vi "TLB Native Dynamic Events ver 0.13e.vi"() -> ()   [LabVIEW 2018]
uses:
  Labview Training Phase 2/Enum Controls/States for Action Engine.ctl
  TLB Type Definitions/State Type Definitions, for 0.26g versions and later 2.ctl
  TLB Type Definitions/Intruction Type Definitions.ctl
  TLB Type Definitions/Encoder cluster.ctl
  TLB Type Definitions/PING CLUSTER.ctl
  <vilib>/Studica/Studica Toolkit/NavX/NavX.lvlib
  <vilib>/Studica/Studica Toolkit/Background/DIO Channel.ctl
  Underlying VI's/NavX VI/navX type def.ctl
  <vilib>/myRIO/Instrument Drivers/Utilities/Utilities.lvlib
  <vilib>/Studica/Studica Toolkit/Background/I2C Channel.ctl
  TLB Type Definitions/Vision cluster.ctl
  <vilib>/NI_Real-Time Target Support.lvlib
  TLB Type Definitions/Stepper cluster.ctl
  Experimental VI's/Archived VI's/MOTOR CONTROL NO PID Type Def.ctl
  Underlying VI's/I2C Master VI/I2C MASTER Type Def.ctl
  Underlying VI's/I2C Master VI/I2C_MASTER_WRITE_NEW Type Def.ctl
  Underlying VI's/Webcam FGV Low level ver/State control.ctl
  <vilib>/userdefined/High Color/IMAQdx.ctl
  Underlying VI's/I2C Master VI/Arduino_Interfacing.ctl
  TLB Type Definitions/Yaw Cluster.ctl
  Experimental VI's/Archived VI's/MOTOR CONTROL NO PID AE DATA ENTRY MODE Type def.ctl
  Experimental VI's/Archived VI's/MOTOR CONTROL NO PID AE DIRECTIONS type def.ctl
  Underlying VI's/Elasped Timer/Control.ctl
  TLB Type Definitions/Time cluster.ctl
  <vilib>/Utility/RT CPU Load.ctl
panel:
  out "Time up flag":bool
  out "Recognized object + Time up?":bool
  out "Speed & distance":T1
  out "Task selection":u8
  out "Object Center Coordinates":cluster{"x":sgl, "y":sgl}
  out "Object detection cluster":T2
  in  "Object recognition mode":enum16{"Ball", "Soap", "Gel", "Pipe", "None"}(ring)
  out "NavX Readings":T3
  out "Arduino Data":T4
  out "CPU loads":T5[](array[typedef]) {"ISR (%)" format="%#.2f"; "Idle (%)" format="%#.2f"; "Background (%)" format="%#.2f"; "Normal (%)" format="%#.2f"; "Above Normal (%)" format="%#.2f"; "High (%)" format="%#.2g"; "Timed Structures (%)" format="%#.2g"; "Time Critical (%)" format="%#.2g"; "Total (%)" format="%#.2g"}
  in  "Red LED":bool
  out "Detect?":bool
  out "TASK ENABLE":bool
  out "Rising Edge":bool
  in  "Green LED":bool
  out "Object detected?":bool
  out "I2C Error":errorcluster
  out "State Logic":T6=enum."Startup"
  out "elements":T7[](array[typedef])
  in  "STOP TASK":bool
  in  "OK Button":bool
  in  "STOP":bool
  out "error out":errorcluster
  out "Action Queue Items":i32
  out "State Logic Queue Items":i32
  out "Action Queues items":string[](array[string])=["Hardware reset", "Software reset", ""]
  out "Action State":string
  # "TLB FRAMEWORK STATUS"
  # "System Health Status Update"
  # "Test Programme written by Calvin Loke    Dated: 28 Aug 2019\nTest Programme revised by Dr Alex See   Dated 30 Aug 2019\n\nProgramme version:   TLB Native Dynamic Events ver 0.04b.vi"
  # "VISION"
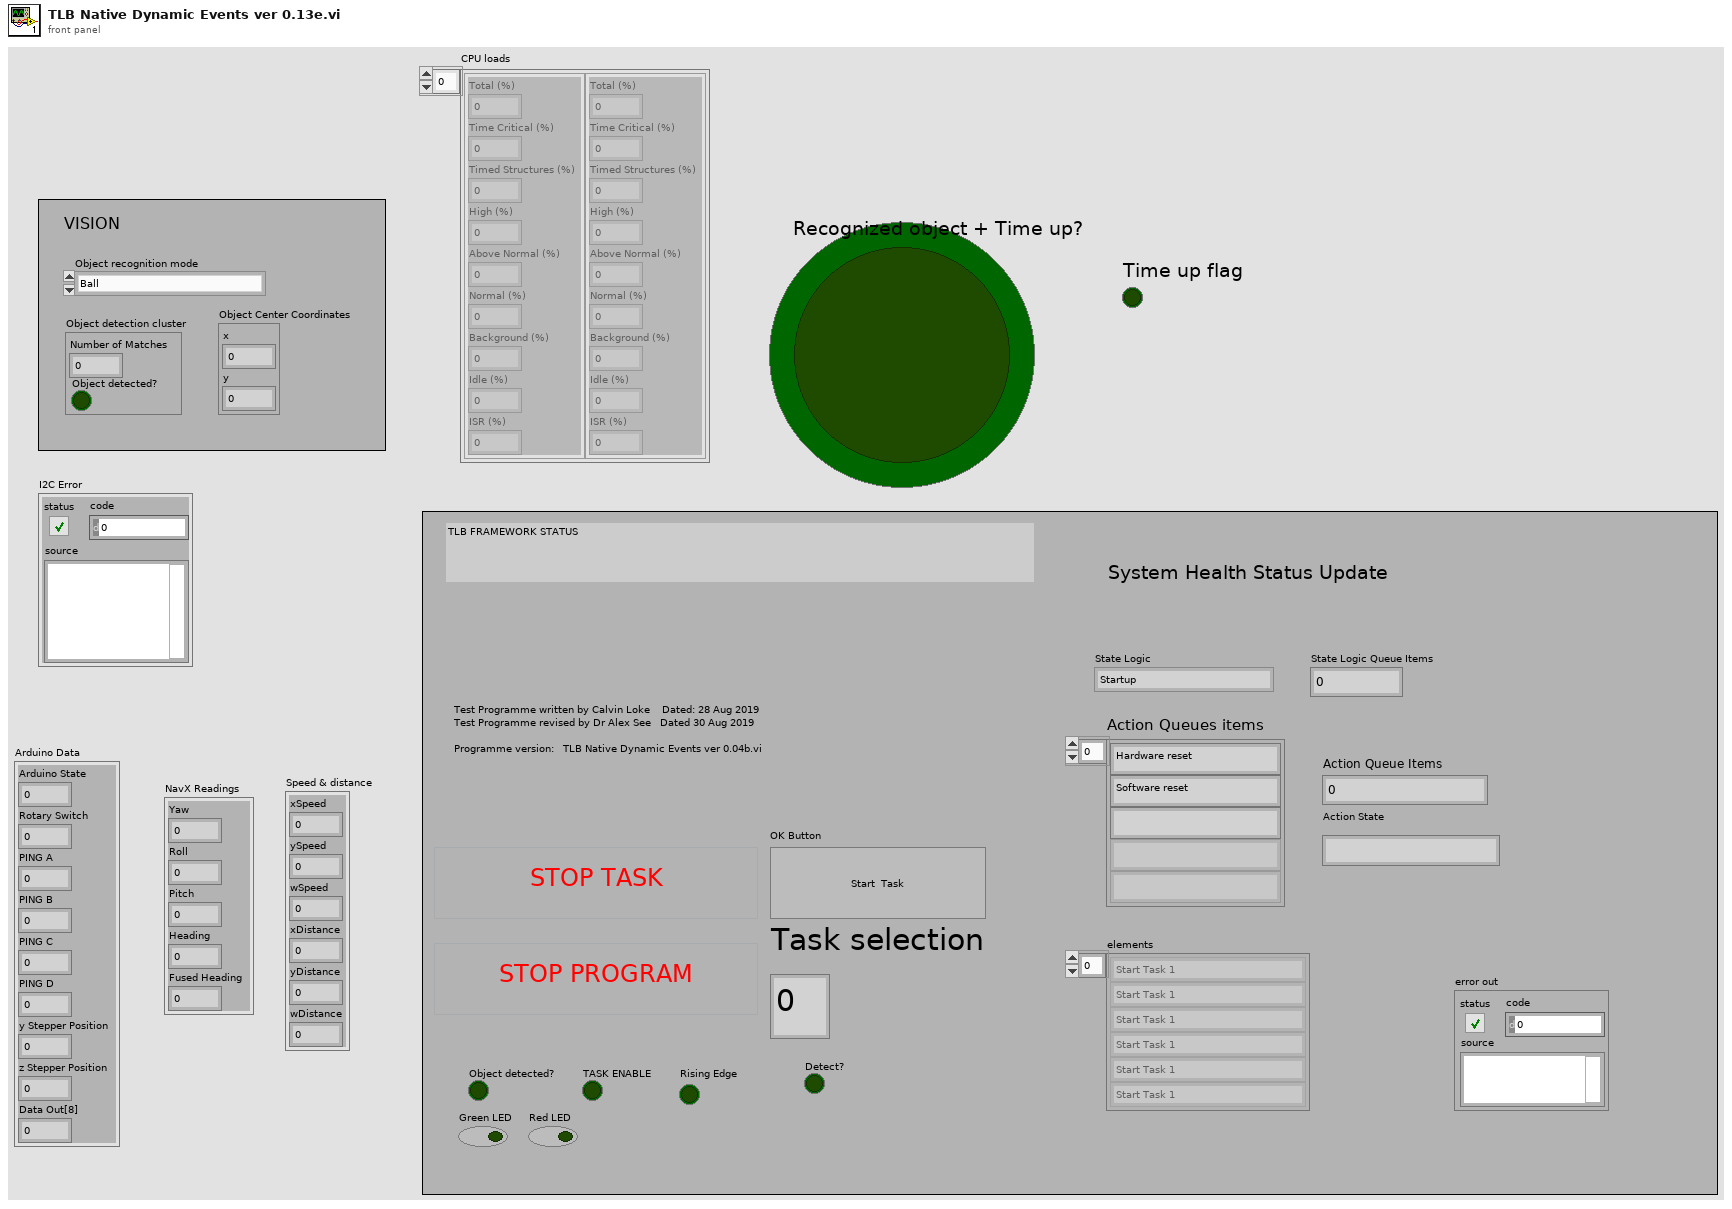
[diagram p1: front panel]
types:
  T1 = cluster{"xSpeed":dbl, "ySpeed":dbl, "wSpeed":dbl, "xDistance":dbl, "yDistance":dbl, "wDistance":dbl}
  T2 = cluster{"Number of Matches":i32, "Object detected?":bool}
  T3 = cluster{"Yaw":dbl, "Roll":dbl, "Pitch":dbl, "Heading":dbl, "Fused Heading":dbl}
  T4 = cluster{"Arduino State":u8, "Rotary Switch":u8, "PING A":u8, "PING B":u8, "PING C":u8, "PING D":u8, "y Stepper Position":u8, "z Stepper Position":u8, "Data Out[8]":u8}
  T5 = typedef "NI_Real-Time Target Support.lvlib/RT CPU Load.ctl" = cluster{"Total (%)":dbl, "Time Critical (%)":dbl, "Timed Structures (%)":dbl, "High (%)":dbl, "Above Normal (%)":dbl, "Normal (%)":dbl, "Background (%)":dbl, "Idle (%)":dbl, "ISR (%)":dbl}
  T6 = typedef "State Type Definitions, for 0.26g versions and later 2.ctl" = enum16{"None", "Startup", "Move to Angle", "True Stop", "Idle", "Shutdown", "Task 1A", "Task 1B", "Task 2:Raise Arm", "Task 2:Sensor Mode", "Task 2:Reverse Mode", "Task 3", "Task 4_A", "Task 4_B", "Task 4_C", "Task 4_D", "Task 5A", "Task 5B", "Task 5C", "Task 5D", "Task 5E: POSITION ARM", "Task 5F: ARM GRAB HEIGHT", "Task 5G: CLOSE CLAW", "Task 5H: RAISE ARM", "Task 6_A", "Task 6_B", "Task 7", "Task 8A: RAISE ARM", "Task 8B: MOVE TO BOX", "Task 8C: CAM BURST", "Task 8D: PROCESS IMAGE", "Task 8E: ROBOT ADJUST", "Task 8F: CAM BURST 2", "Task 8G: PROCESS IMAGE 2", "Task 8H: ARM ADJUST", "Task 8I: ARM GRAB HEIGHT", "Task 8J: CLOSE CLAW", "Task 8K: RAISE MY SWORD", "Task 9A: Raise Arm", "Task 9B: Rotate to Angle", "Task 9C: Detect Box", "Task 9D: MOVE FORWARD", "Task 9E: MOVE LEFT", "Task 9F: SCAN BOX", "Task 9G: MOVE RIGHT", "Task 9H: SCAN BOX 2", "Task 9I: ROTATE 90 CW", "Task 9J: FORWARD", "Task 9K: MOVE RIGHT", "Task 9L: SCAN BOX 3", "Task 9M: MOVE RIGHT", "Task 9N: SCAN BOX 4", "PENIS", "PENIS 2", "PENIS 3", "Task 9R: PROCESS COLOUR", "Task A1: Task 9 Open cam", "Task A2: Task 9 Move Arm", "Task A3: Task 9 Set Timer", "Task A4: Tasl 9 Capture images", "Task A5: Task 9 Close camera", "Task A6: Process Colour", "Task A7: Dispose Camera Buffer"}
  T7 = typedef "Intruction Type Definitions.ctl" = enum16{"None", "Start Task 1", "Start Task 2", "Start Task 3", "Start Task 4", "Start Task 5", "Start Task 6", "Start Task 7", "Start Task 8 - BALL", "Start Task 8 - Gel", "Start Task 8 - Pipe", "Start Task 8 - Soap", "Start Task 9", "Start Task A", "Start Task B", "Exit"}
  T8 = typedef "Time cluster.ctl" = cluster{"Time up flag":bool, "SET TIME TO CHECK":dbl}
  T9 = typedef "Yaw Cluster.ctl" = cluster{"Yaw":dbl, "Compass":dbl}
  T10 = typedef "Stepper cluster.ctl" = cluster{"y Stepper Position":u8, "z Stepper Position":u8}
  T11 = typedef "DIO Channel.ctl" = enum16{"Not Connected", "A/DIO1", "A/DIO2", "A/DIO3", "A/DIO4", "A/DIO5", "A/DIO6", "A/DIO7", "A/DIO13", "B/DIO1", "B/DIO2", "B/DIO3", "B/DIO4", "B/DIO5", "B/DIO6", "B/DIO7", "B/DIO13", "C/DIO0", "C/DIO1", "C/DIO2", "C/DIO3", "C/DIO4", "C/DIO5", "C/DIO6", "C/DIO7"}
  T12 = typedef "Vision cluster.ctl" = cluster{"Recognized Object":bool, "Object X coordinate":dbl, "Object Y coordinate":dbl}
  T13 = typedef "PING CLUSTER.ctl" = cluster{"PING_A":u8, "PING_B":u8, "PING_C":u8, "PING_D":u8}
  T14 = typedef "Encoder cluster.ctl" = cluster{"xDistance":dbl, "yDistance":dbl, "wDistance":dbl}
  T15 = cluster{"DIO Channel":T11, "FPGA VI Reference Out":refnum<k20>}
  T16 = typedef "MOTOR CONTROL NO PID AE DATA ENTRY MODE Type def.ctl" = enum16{"Initialize", "Reset Encoders", "Write to motors", "Read from Encoders"}
  T17 = typedef "navX type def.ctl" = enum16{"Get i2C reference", "Read Values", "Zero Yaw"}
  T18 = typedef "Arduino_Interfacing.ctl" = enum16{"Initialize", "Write to Arduino", "Read From Arduino"}
  T19 = typedef "I2C Channel.ctl" = enum16{"Not Connected", "A", "B"}
  T20 = typedef "States for Action Engine.ctl" = enum16{"Initialize", "Write", "Read"}
  T21 = cluster{"I2C Ref Out":cluster{"I2C Channel":T19, "FPGA VI Reference Out":refnum<k20>}, "Connected":bool, "Slave Address (7-bit)":u8, "Registry":u8[]}
  T22 = typedef "IMAQ Image.ctl" = refnum<image>
  T23 = typedef "State Type Definitions.ctl" = enum16{"None", "Startup", "Move to Angle", "True Stop", "Idle", "Shutdown", "Task 1", "Task 2:Raise Arm", "Task 2:Sensor Mode", "Task 2:Reverse Mode", "Task 3", "Task 4_A", "Task 4_B", "Task 4_C", "Task 4_D", "Task 5A: ARM CAM HEIGHT", "Task 5B: MOVE TO BOX", "Task 5C: CAM BURST", "Task 5D: PROCESS IMAGE", "Task 5E: POSITION ARM", "Task 5F: ARM GRAB HEIGHT", "Task 5G: CLOSE CLAW", "Task 5H: RAISE ARM", "Task 6_A", "Task 6_B", "Task 7", "Task 8A: RAISE ARM", "Task 8B: MOVE TO BOX", "Task 8C: CAM BURST", "Task 8D: PROCESS IMAGE", "Task 8E: ROBOT ADJUST", "Task 8F: CAM BURST 2", "Task 8G: PROCESS IMAGE 2", "Task 8H: ARM ADJUST", "Task 8I: ARM GRAB HEIGHT", "Task 8J: CLOSE CLAW", "Task 8K: RAISE MY SWORD", "Task 9A: Raise Arm", "Task 9B: Rotate to Angle", "Task 9C: Detect Box", "Task 9D: MOVE FORWARD", "Task 9E: MOVE LEFT", "Task 9F: SCAN IMAGE", "Task 9G: PROCESS COLOUR", "Task 9H: MOVE RIGHT", "Task 9I: SCAN IMAGE", "Task 9J: PROCESS COLOUR", "Task 9K: ROTATE 90 CW", "Task 9L: MOVE FORWARD", "Task 9M: MOVE RIGHT", "Task 9N: SCAN IMAGE", "Task 9O: PROCESS COLOUR", "Task 9P: MOVE RIGHT", "Task 9Q: SCAN IMAGE", "Task 9R: PROCESS COLOUR"}
  T24 = typedef "State Type Definitions.ctl" = enum16{"None", "Startup", "Move to Angle", "True Stop", "Idle", "Shutdown", "Task 1", "Task 2", "Task 3", "Task 4_A", "Task 4_B", "Task 4_C", "Task 5_A", "Task 5 _B", "Task 5_C", "Task 6_A", "Task 6_B", "Task 7", "Task 8", "Task 9", "Task A", "Task B"}
  T25 = typedef "MOTOR CONTROL NO PID AE DIRECTIONS type def.ctl" = enum16{"y-axis movement", "x-axis movement", "Rotate", "Stop"}
  T26 = typedef "Control.ctl" = enum16{"Start", "Pause", "Initialize"}
  T27 = typedef "I2C_MASTER_WRITE_NEW Type Def.ctl" = enum16{"Ultrasonic sensors", "Stepper origin", "zStepper 13.3k", "zStepper 13k", "zStepper 12k", "zStepper 11k", "zStepper 10k", "zStepper 9k", "zStepper 8k", "zStepper 7k", "zStepper 6k", "zStepper 5k", "zStepper 4k", "zStepper 3k", "zStepper 2k", "zStepper 1k", "zStepper 900", "zStepper 800", "zStepper 700", "zStepper 600", "zStepper 500", "zStepper 400", "zStepper 300", "zStepper 200", "zStepper 100", "zStepper 0", "yStepper control", "Open Claw", "Close Claw", "Soft Reset"}
  T28 = typedef "State control.ctl" = enum16{"Initialise", "Start camera", "Continuous Acquisition ", "Stop camera", "Dispose all"}
  T29 = typedef "IMAQdx.ctl" = refnum<k21>
  T30 = typedef "MOTOR CONTROL NO PID Type Def.ctl" = enum16{"Init", "Front Back", "Left Right", "Rotate", "Stop", "Latch"}
  T31 = typedef "I2C MASTER Type Def.ctl" = enum16{"Last State", "Mode 0", "Mode 1", "Mode 2", "Mode 3", "Mode 4", "Mode 5", "Mode 6", "Mode 7", "Mode 8", "Mode 9", "Mode 10"}
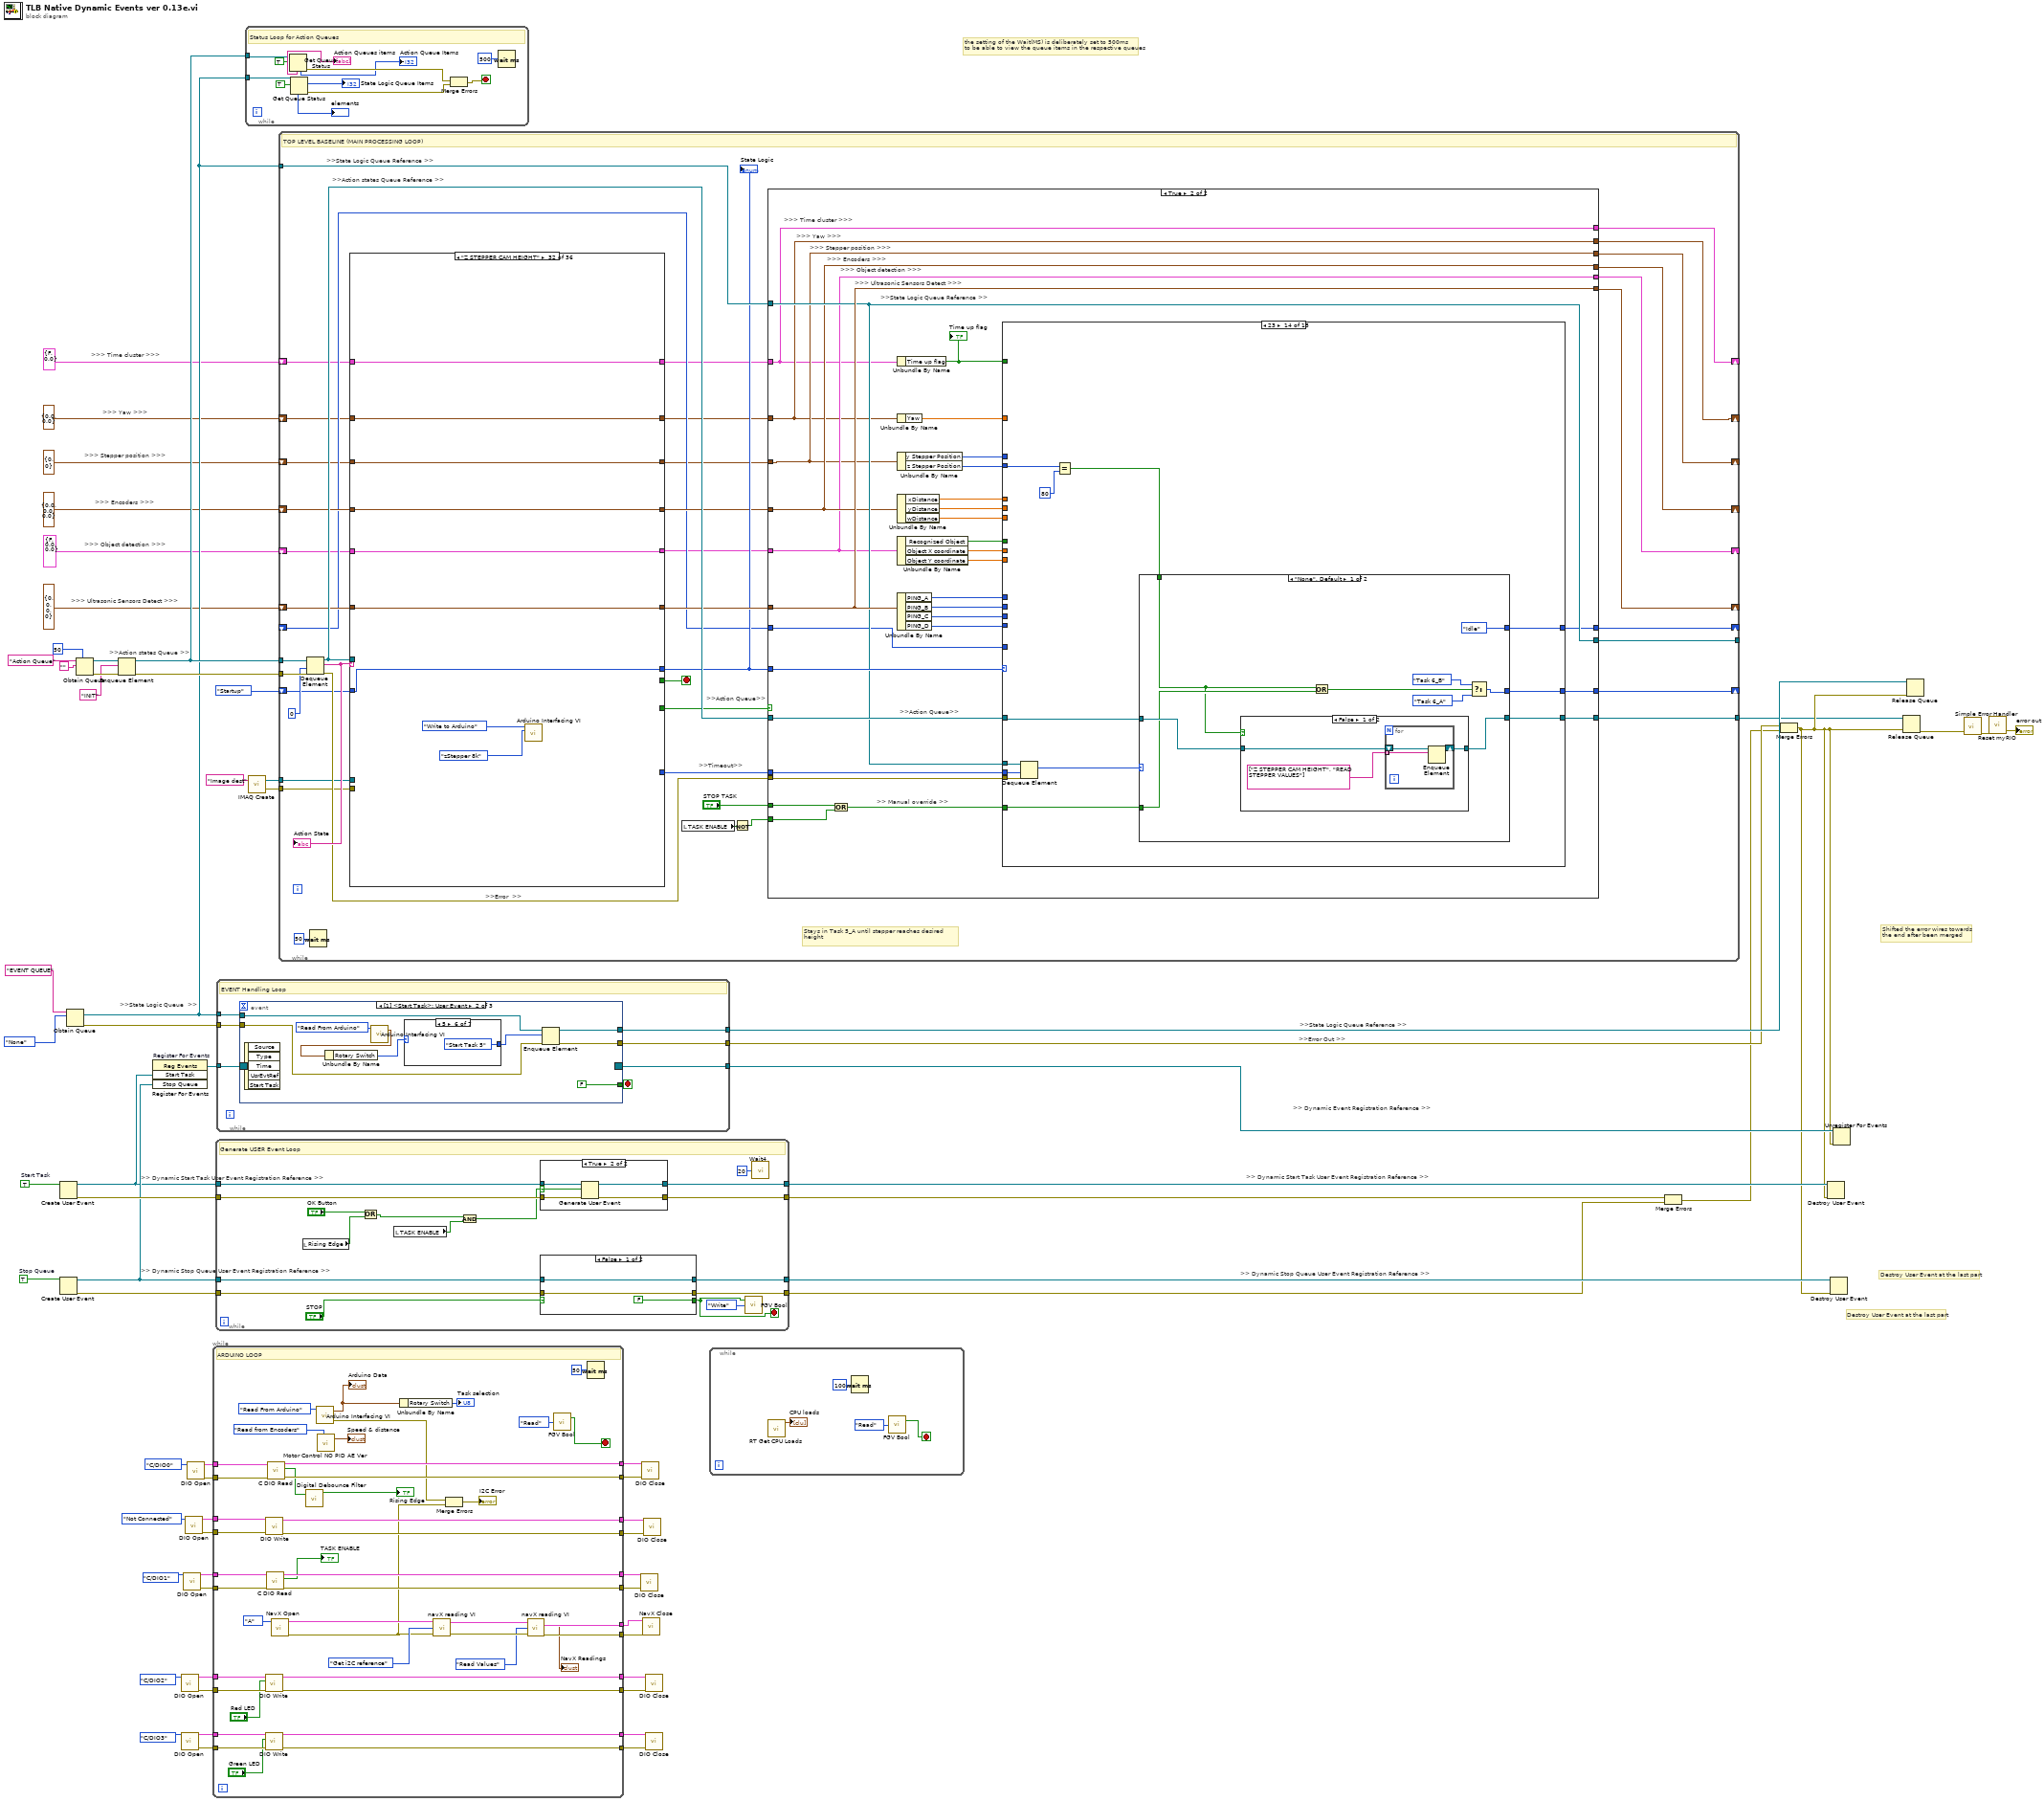
[diagram p0: block diagram]
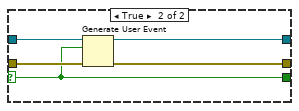
[diagram p2: hidden frame]
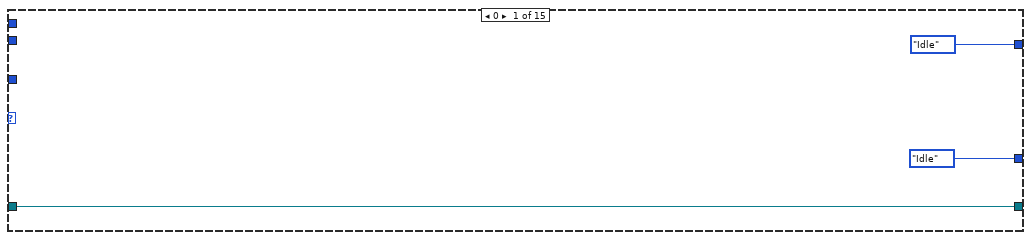
[diagram p5: hidden frame]
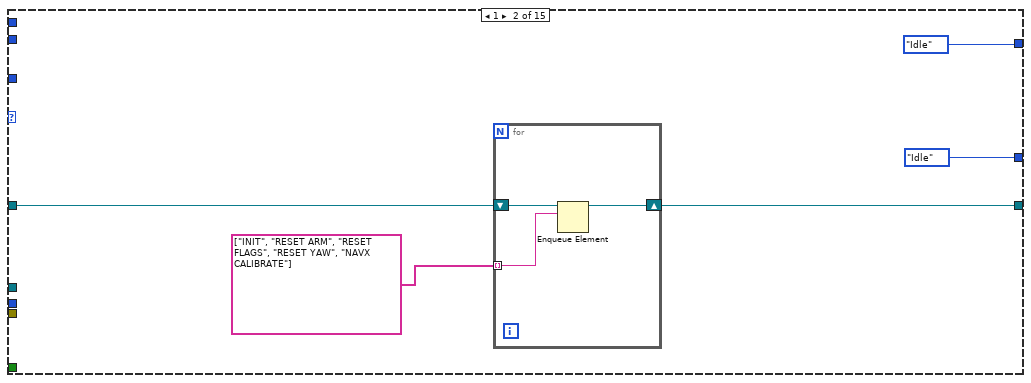
[diagram p6: hidden frame]
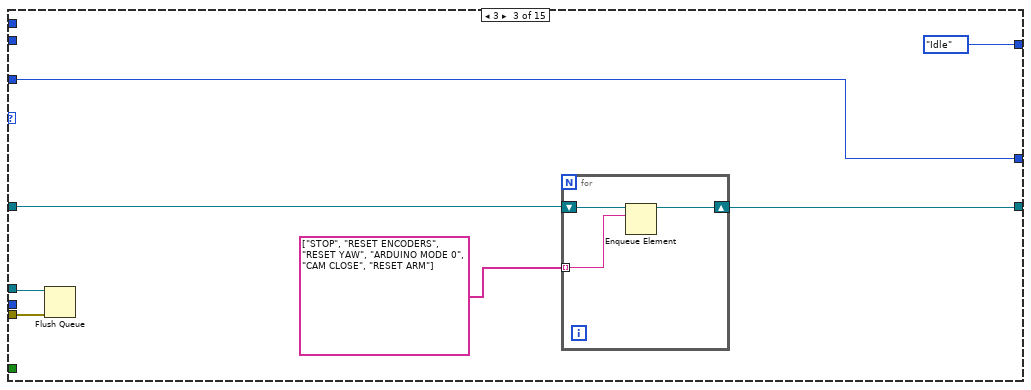
[diagram p7: hidden frame]
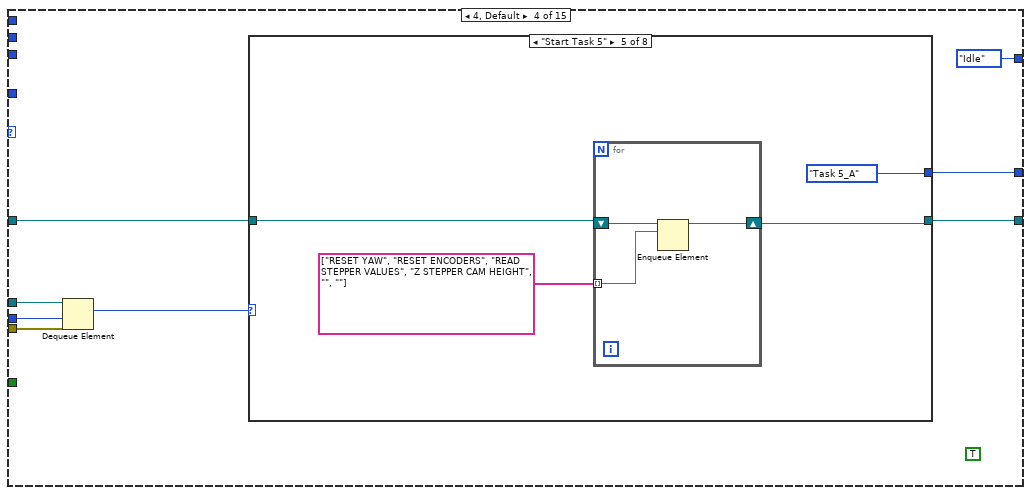
[diagram p8: hidden frame]
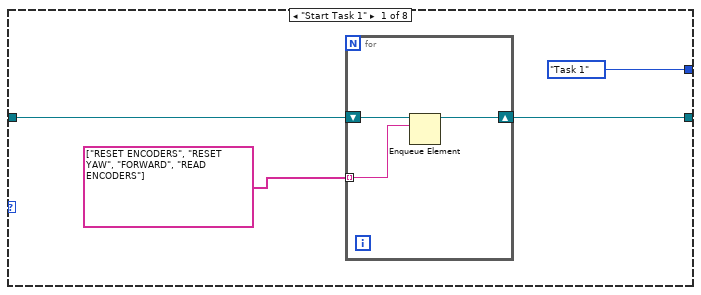
[diagram p9: hidden frame]
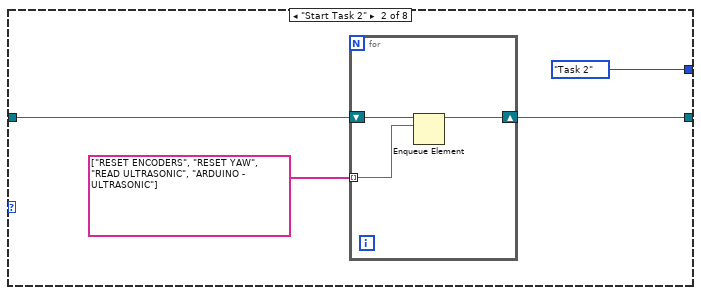
[diagram p10: hidden frame]
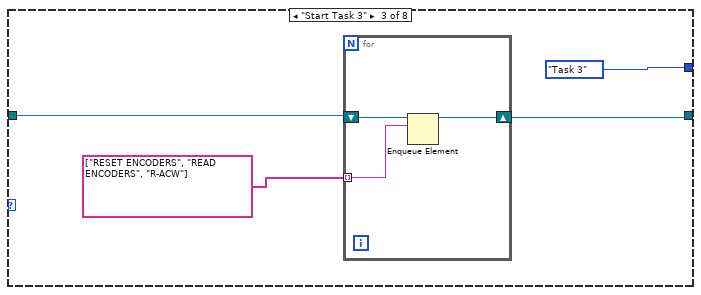
[diagram p11: hidden frame]
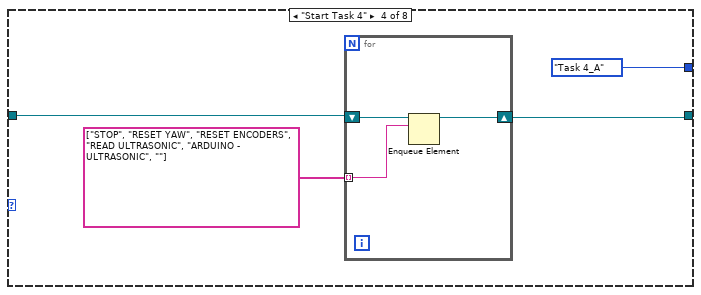
[diagram p12: hidden frame]
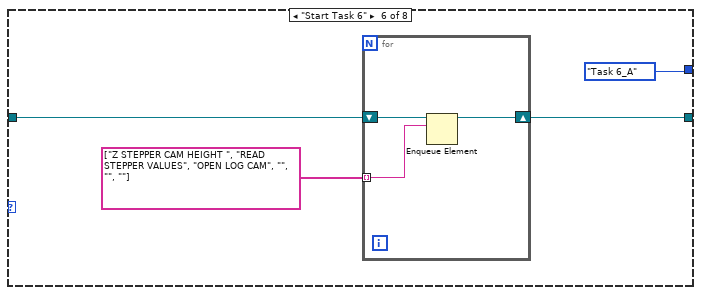
[diagram p13: hidden frame]
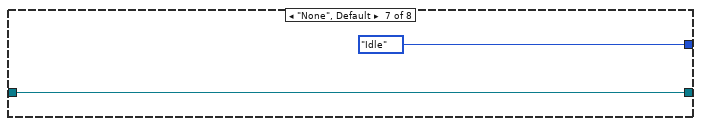
[diagram p14: hidden frame]
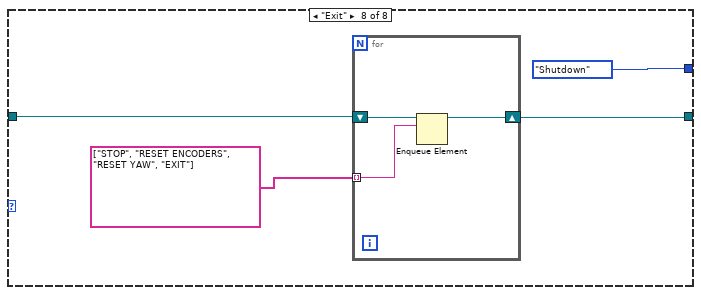
[diagram p15: hidden frame]
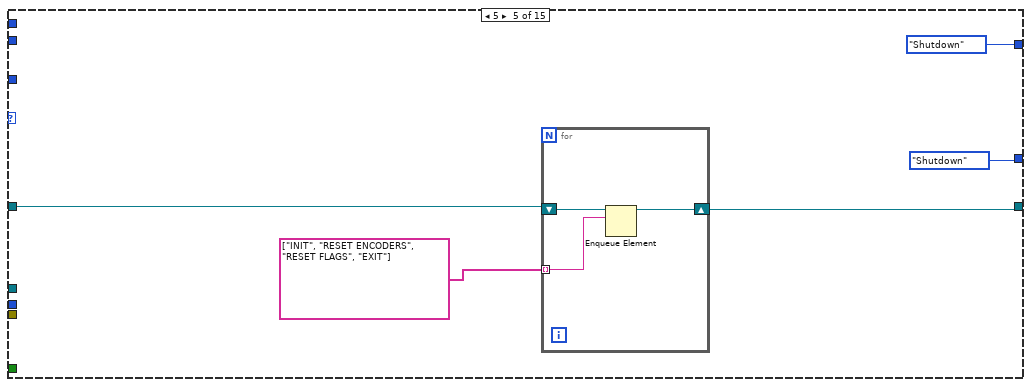
[diagram p16: hidden frame]
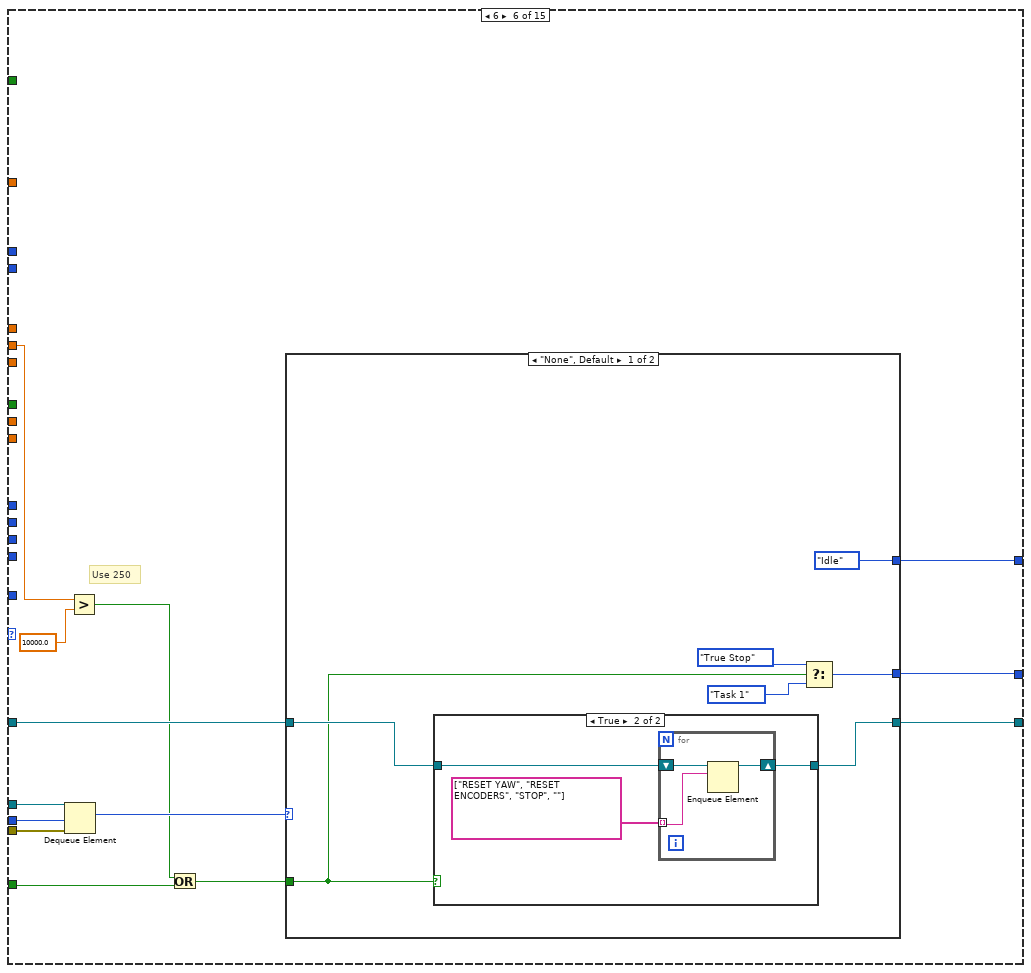
[diagram p17: hidden frame]
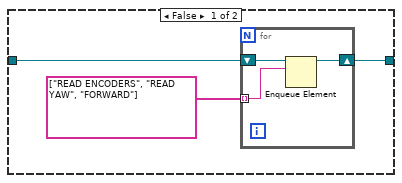
[diagram p18: hidden frame]
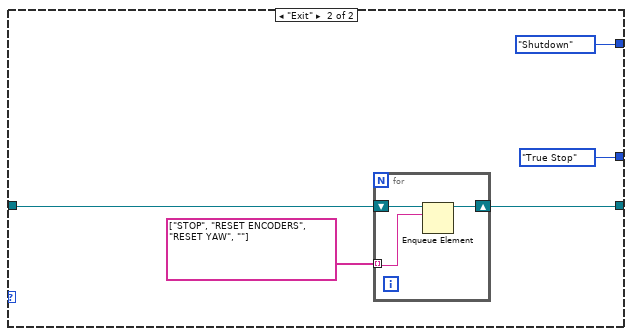
[diagram p19: hidden frame]
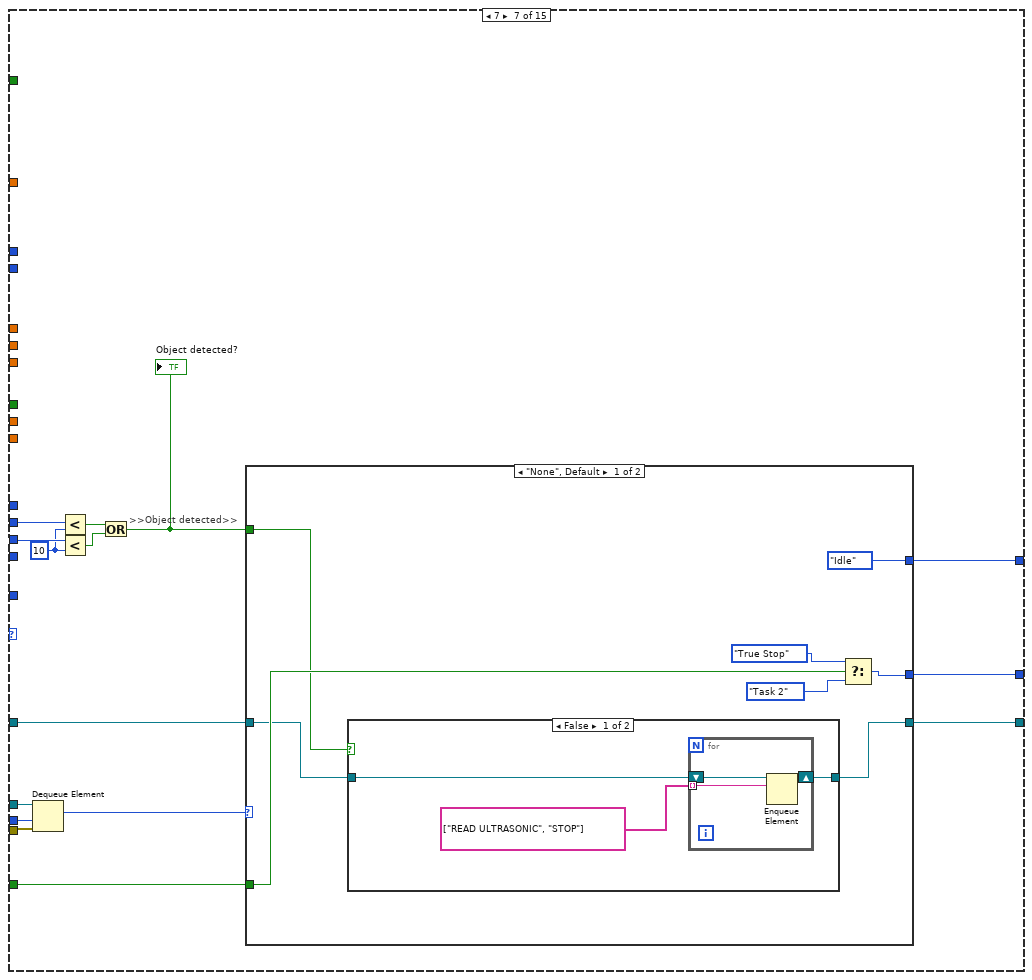
[diagram p20: hidden frame]
diagram:
  w69 = TRUE  # Stop Queue
  w68 = TRUE  # Start Task
  # ">>> Time cluster >>>"
  # ">>> Yaw >>>"
  # ">>> Stepper position >>>"
  # ">>> Encoders >>>"
  # ">>> Object detection >>>"
  # ">>> Ultrasonic Sensors Detect >>>"
  # "the setting of the Wait(MS) is deliberately set to 500ms\nto be able to view the queue items in the respective queues"
  # ">>Error Out >>"
  # ">> Dynamic Stop Queue User Event Registration Reference >>"
  # ">> Dynamic Start Task User Event Registration Reference >>"
  # ">> Dynamic Stop Queue User Event Registration Reference >>"
  # ">> Dynamic Start Task User Event Registration Reference >>"
  # ">> Dynamic Event Registration Reference >>"
  # ">>Action states Queue >>"
  # ">>State Logic Queue  >>"
  # ">>State Logic Queue Reference >>"
  # "Destroy User Event at the last part"
  # "Destroy User Event at the last part"
  # "Shifted the error wires towards\nthe end after been merged"
  n1 = Create User Event(user event datatype=w68) -> (user event=w60:refnum<user-event>, error out=w65:errorcluster)  [unwired: 1 in]
  n2 = Create User Event(user event datatype=w69) -> (user event=w61:refnum<user-event>, error out=w64:errorcluster)  [unwired: 1 in]
  n3 = Obtain Queue(name (unnamed)="EVENT QUEUE", element data type=Intruction_Type_Definitions."None" ("Enum")) -> (queue out=w46:refnum<queue>, error out=w52:errorcluster)  [unwired: 3 in, 1 out]
  n4 = Obtain Queue(max queue size (-1, unlimited)=50, name (unnamed)="Action Queue", element data type="") -> (queue out=w55:refnum<queue>, error out=w51:errorcluster)  [unwired: 2 in, 1 out]
  n5 = Enqueue Element(queue=w55, element="INIT", error in (no error)=w51) -> (queue out=w47:refnum<queue>, error out=w50:errorcluster)  [unwired: 1 in, 1 out]
  n6 = register-events "Register For Events"(w60, w61) -> (reference out=w59:refnum<event-registration>)  [unwired: 2 in, 1 out]
  n7 = call <vilib>:"DIO Open.vi"("DIO Channel"=DIO_Channel."C/DIO2") -> ("error out"=w13:errorcluster, "DIO Info Out"=w14:T15)  [unwired: 9 in]
  n8 = call <vilib>:"DIO Open.vi"("DIO Channel"=DIO_Channel."C/DIO3") -> ("error out"=w8:errorcluster, "DIO Info Out"=w9:T15)  [unwired: 9 in]
  n9 = call <vilib>:"DIO Open.vi"("DIO Channel"=DIO_Channel."C/DIO1") -> ("error out"=w24:errorcluster, "DIO Info Out"=w25:T15)  [unwired: 9 in]
  n10 = call <vilib>:"DIO Open.vi"("DIO Channel"=DIO_Channel."Not Connected") -> ("error out"=w29:errorcluster, "DIO Info Out"=w31:T15)  [unwired: 9 in]
  n11 = call <vilib>:"DIO Open.vi"("DIO Channel"=DIO_Channel."C/DIO0") -> ("error out"=w34:errorcluster, "DIO Info Out"=w37:T15)  [unwired: 9 in]
  n12 = while {
    tunnel: w37 -> [w111]
    tunnel: [w110] -> w35
    tunnel: w34 -> [w109]
    tunnel: [w108] -> w33
    tunnel: w31 -> [w104]
    tunnel: [w103] -> w30
    tunnel: w29 -> [w102]
    tunnel: [w101] -> w28
    tunnel: [w100] -> w26
    tunnel: w25 -> [w99]
    tunnel: w24 -> [w98]
    tunnel: [w97] -> w23
    tunnel: w14 -> [w91]
    tunnel: w13 -> [w90]
    tunnel: [w89] -> w12
    tunnel: [w88] -> w11
    tunnel: w9 -> [w86]
    tunnel: w8 -> [w85]
    tunnel: [w84] -> w7
    tunnel: [w83] -> w6
    tunnel: [w77] -> w3
    tunnel: [w76] -> w4
    stop <- w113 stop-if-true
    # "ARDUINO LOOP"
    n13 = call <vilib>:"DIO Write.vi"("error in (no error)"=w90, "Input"="Red LED", "DIO Info In"=w91) -> ("error out"=w88:errorcluster, "DIO Info Out"=w89:T15)  [unwired: 7 in]
    n14 = call <vilib>:"DIO Write.vi"("error in (no error)"=w85, "Input"="Green LED", "DIO Info In"=w86) -> ("error out"=w83:errorcluster, "DIO Info Out"=w84:T15)  [unwired: 7 in]
    n15 = call <vilib>:"DIO Write.vi"("error in (no error)"=w102, "DIO Info In"=w104) -> ("error out"=w101:errorcluster, "DIO Info Out"=w103:T15)  [unwired: 8 in]
    n16 = call <vilib>:"C DIO Read.vi"("error in (no error)"=w98, "DIO Info In in"=w99) -> ("error out"=w97:errorcluster, "IN"=→"TASK ENABLE":bool, "DIO Info In out"=w100:T15)  [unwired: 7 in]
    n17 = call <vilib>:"C DIO Read.vi"("error in (no error)"=w109, "DIO Info In in"=w111) -> ("error out"=w108:errorcluster, "IN"=w106:bool, "DIO Info In out"=w110:T15)  [unwired: 7 in]
    n18 = call <vilib>:"NavX Open.vi"("I2C Channel"=I2C_Channel."A") -> ("error out"=w93:errorcluster, "NavX Info"=w95:T21)  [unwired: 9 in]
    n19 = call "Digital Debounce Filter.vi"("Boolean input"=w106) -> ("Rising Edge"=→"Rising Edge":bool)  [unwired: 1 in, 2 out]
    n20 = call "Arduino Interfacing VI.vi"("AE Mode"=Arduino_Interfacing."Read From Arduino") -> ("error out"=w80:errorcluster, "Arduino Data"=w73:T4)  [unwired: 3 in]
    "Arduino Data" <- w73
    n21 = call "Motor Control NO PID AE Ver.vi"("AE Mode"=MOTOR_CONTROL_NO_PID_AE_DATA_ENTRY_MODE_Type_def."Read from Encoders") -> ("Speed & distance"=→"Speed & distance":T1)  [unwired: 4 in, 1 out]
    n22 = Unbundle By Name(w73) -> ("Rotary Switch"=→"Task selection":u8)
    n23 = call "navX reading VI.vi"("NavX Info In"=w95, "Mode"=navX_type_def."Get i2C reference", "error in (no error)"=w93) -> ("NavX Info Out"=w79:T21, "Error Out"=w78:errorcluster)  [unwired: 2 out]
    n24 = Merge Errors(w80, w93) -> (→"I2C Error":errorcluster)
    n25 = call "navX reading VI.vi"("NavX Info In"=w79, "Mode"=navX_type_def."Read Values", "error in (no error)"=w78) -> ("NavX Info Out"=w77:T21, "NavX Readings"=→"NavX Readings":T3, "Error Out"=w76:errorcluster)  [unwired: 1 out]
    n26 = call "FGV Bool.vi"("Init/Read/Write State"=States_for_Action_Engine."Read") -> ("Output node"=w113:bool)  [unwired: 2 in, 1 out]
    n27 = Wait (ms)(milliseconds to wait=u32 50) -> ()  [unwired: 1 out]
  }
  n28 = while {
    tunnel: w60 -> [w131]
    tunnel: w61 -> [w130]
    tunnel: [w129] -> w67
    tunnel: [w128] -> w66
    tunnel: w65 -> [w127]
    tunnel: [w126] -> w63
    tunnel: w64 -> [w125]
    tunnel: [w124] -> w62
    stop <- w122 stop-if-true
    # "Generate USER Event Loop"
    n29 = local read "Rising Edge"() -> (w118:bool)
    n30 = Or(x="OK Button", y=w118) -> (x .or. y?=w117:bool)
    n31 = local read "TASK ENABLE"() -> (w116:bool)
    n32 = And(x=w117, y=w116) -> (x .and. y?=w115:bool)
    n33 = case shown="True" w115 {
      selector: w115 -> [_ w142]
      tunnel: w131 -> [w141 w146]
      tunnel: [w141 w145] -> w128
      tunnel: w127 -> [w140 w144]
      tunnel: [w140 w143] -> w126
      frame False {
      }
      frame True {
        n34 = Generate User Event(user event=w146, event data cluster=w142, error in=w144) -> (user event out=w145:refnum<user-event>, error out=w143:errorcluster)  [unwired: 1 in]
      }
    }
    n35 = case shown="False" "STOP" {
      selector: "STOP" -> [_ w135]
      tunnel: w130 -> [w134 w139]
      tunnel: [w134 w138] -> w129
      tunnel: w125 -> [w133 w137]
      tunnel: [w133 w136] -> w124
      tunnel: [FALSE w135] -> w122
      frame False {
      }
      frame True {
        n36 = Generate User Event(user event=w139, event data cluster=w135, error in=w137) -> (user event out=w138:refnum<user-event>, error out=w136:errorcluster)  [unwired: 1 in]
      }
    }
    n37 = call "FGV Bool.vi"("Init/Read/Write State"=States_for_Action_Engine."Write", "Input Node"=w122) -> ()  [unwired: 1 in, 2 out]
    n38 = call "Wait4"("Count(uSec)"=u32 20) -> ()  [unwired: 1 out]
  }
  n39 = while {
    tunnel: w59 -> [w153]
    tunnel: [w152] -> w58
    tunnel: w46 -> [w150]
    tunnel: [w149] -> w57
    tunnel: w52 -> [w148]
    tunnel: [w147] -> w49
    stop <- w151 stop-if-true
    # "EVENT Handling Loop"
    n40 = event shown="[1] <Start Task>: User Event" {
      selector: w153 -> [_ _ _]
      dyn-events: [_ _ _] -> w152
      timeout: _ -> [_ _ _]
      tunnel: [FALSE FALSE w181] -> w151
      tunnel: w150 -> [w158 w167 w179]
      tunnel: [w157 w166 w180] -> w149
      tunnel: w148 -> [w156 w165 w178]
      tunnel: [w155 w164 w177] -> w147
      event Timeout {
        n41 = event-data() -> ()  [unwired: 1 in, 3 out]
        n42 = Enqueue Element(queue=w158, element=Intruction_Type_Definitions."None" ("Enum"), error in (no error)=w156) -> (queue out=w157:refnum<queue>, error out=w155:errorcluster)  [unwired: 1 in, 1 out]
      }
      event User Event {
        n43 = event-data() -> ()  [unwired: 1 in, 5 out]
        n44 = call "Arduino Interfacing VI.vi"("AE Mode"=Arduino_Interfacing."Read From Arduino") -> ("Arduino Data"=w161:T4)  [unwired: 3 in, 1 out]
        n45 = Unbundle By Name(w161) -> ("Rotary Switch"=w160:u8)
        n46 = case shown="5" w160 {
          tunnel: [Intruction_Type_Definitions."None" ("Enum") Intruction_Type_Definitions."Start Task 1" ("Enum") Intruction_Type_Definitions."Start Task 2" ("Enum") Intruction_Type_Definitions."Start Task 3" ("Enum") Intruction_Type_Definitions."Start Task 4" ("Enum") Intruction_Type_Definitions."Start Task 5" ("Enum") Intruction_Type_Definitions."Start Task 6" ("Enum")] -> w163
          frame 0, Default {
          }
          frame 1 {
          }
          frame 2 {
          }
          frame 3 {
          }
          frame 4 {
          }
          frame 5 {
          }
          frame 6 {
          }
        }
        n47 = Enqueue Element(queue=w167, element=w163, error in (no error)=w165) -> (queue out=w166:refnum<queue>, error out=w164:errorcluster)  [unwired: 1 in, 1 out]
      }
      event User Event {
        n48 = event-data() -> ("Stop Queue"=w181:bool)  [unwired: 1 in, 4 out]
        n49 = Enqueue Element At Opposite End(queue=w179, element=Intruction_Type_Definitions."Exit" ("Enum"), error in (no error)=w178) -> (queue out=w180:refnum<queue>, error out=w177:errorcluster)  [unwired: 1 in, 1 out]
      }
    }
  }
  n50 = while {
    tunnel: w47 -> [w191]
    tunnel: w46 -> [w188]
    stop <- w185 stop-if-true
    # "Status Loop for Action Queues"
    n51 = Get Queue Status(queue=w191, return elements? (F)=TRUE) -> (error out=w187:errorcluster, # elements in queue=→"Action Queue Items":i32, elements=→"Action Queues items":string[])  [unwired: 1 in, 5 out]
    n52 = Get Queue Status(queue=w188, return elements? (F)=TRUE) -> (# pending remove=→"State Logic Queue Items":i32, error out=w186:errorcluster, elements=→"elements":T7[])  [unwired: 1 in, 5 out]
    n53 = Merge Errors(w187, w186) -> (w185:errorcluster)
    n54 = Wait (ms)(milliseconds to wait=u32 500) -> ()  [unwired: 1 out]
  }
  n55 = call "IMAQ Create"("Image Name"="Image dest") -> ("New Image"=w18:T22, "error out"=w17:errorcluster)  [unwired: 4 in]
  n56 = while {
    tunnel: w46 -> [w222]
    tunnel: w47 -> [w234]
    tunnel: w50 -> [w232]
    tunnel: [w231] -> _
    tunnel: [w230] -> w40
    shift-right: [w223] -> _
    shift-left: T13 {"PING_A"=0, "PING_B"=0, "PING_C"=0, "PING_D"=0} -> [w225]
    shift-right: [w216] -> _
    shift-left: State_Type_Definitions,_for_0.26g_versions_and_later_2."Startup" ("Enum") -> [w219]
    shift-right: [w212] -> _
    shift-left: T14 {"xDistance"=0.0, "yDistance"=0.0, "wDistance"=0.0} -> [w214]
    shift-right: [w209] -> _
    shift-left: _ -> [w208]
    tunnel: w18 -> [w207]
    tunnel: w17 -> [w206]
    shift-right: [w203] -> _
    shift-left: T12 {"Recognized Object"=FALSE, "Object X coordinate"=0.0, "Object Y coordinate"=0.0} -> [w205]
    shift-right: [w200] -> _
    shift-left: T10 {"y Stepper Position"=0, "z Stepper Position"=0} -> [w202]
    shift-right: [w197] -> _
    shift-left: T9 {"Yaw"=0.0, "Compass"=0.0} -> [w199]
    shift-right: [w194] -> _
    shift-left: T8 {"Time up flag"=FALSE, "SET TIME TO CHECK"=0.0} -> [w196]
    stop <- w221 stop-if-true
    # "Stays in Task 5_A until stepper reaches desired \nheight"
    # ">>Error  >>"
    # ">>Action Queue>>"
    # ">>Timeout>>"
    # ">>Action states Queue Reference >>"
    # ">>State Logic Queue Reference >>"
    # "TOP LEVEL BASELINE (MAIN PROCESSING LOOP)"
    n57 = Dequeue Element(queue=w234, timeout in ms (-1)=0, error in (no error)=w232) -> (queue out=w226:refnum<queue>, element=w233:string, error out=w227:errorcluster)  [unwired: 1 out]
    "Action State" <- w233
    n58 = Wait (ms)(milliseconds to wait=u32 50) -> ()  [unwired: 1 out]
    n59 = case shown="\"Z STEPPER CAM HEIGHT\"" w233 {
      tunnel: [_ _ _ _ _ _ _ _ _ _ _ _ _ _ _ _ 0 w991 _ _ _ _ _ _ _ _ _ _ _ _ _ _ _ _ _ _] -> w229
      tunnel: w226 -> [_ _ _ _ _ _ _ _ _ _ _ _ _ _ _ _ _ _ _ _ _ _ _ _ _ _ _ _ _ _ _ _ _ _ _ _]
      tunnel: w225 -> [w807 w815 w826 w837 w847 w857 w868 w879 w889 w895 w909 w922 w932 w940 w964 w973 w983 w992 w1000 w1008 w1037 w1047 w1054 w1062 w1074 w1086 w1105 w1116 w1122 w1131 w1140 w1149 w1161 w1166 w1177 w1187]
      tunnel: [w807 w815 w826 w837 w847 w857 w868 w879 w889 w895 w909 w923 w932 w940 w965 w973 w983 w992 w1000 w1008 w1036 w1047 w1054 w1062 w1074 w1086 w1105 w1116 w1122 w1131 w1140 w1149 w1161 w1166 w1177 w1187] -> w224
      tunnel: [TRUE TRUE _ _ _ _ _ _ _ _ _ _ _ _ _ _ _ _ _ _ _ _ _ _ _ _ _ _ _ _ _ _ _ _ _ _] -> w221
      tunnel: w219 -> [w805 w813 w825 w836 w846 w856 w867 w878 w888 w894 w908 w921 w931 w939 w963 w972 w980 w989 w999 w1007 w1035 w1046 w1053 w1061 w1068 w1080 w1104 w1111 w1121 w1130 w1139 w1148 w1160 w1165 w1176 w1186]
      tunnel: [_ _ _ _ _ _ _ _ _ _ _ _ _ _ _ _ _ TRUE _ _ _ _ _ _ _ _ _ _ _ _ _ _ _ _ _ _] -> w218
      tunnel: [w805 w813 w825 w836 w846 w856 w867 w878 w888 w894 w908 w921 w931 w939 w963 w972 w980 w989 w999 w1007 w1035 w1046 w1053 w1061 w1068 w1080 w1104 w1111 w1121 w1130 w1139 w1148 w1160 w1165 w1176 w1186] -> w217
      tunnel: w214 -> [w804 w812 w824 w835 w845 w855 w866 w877 w887 w896 w907 w920 w933 w941 w962 w974 w979 w988 w1001 w1009 w1025 w1045 w1056 w1063 w1075 w1087 w1106 w1117 w1124 w1133 w1142 w1151 w1163 w1168 w1179 w1189]
      tunnel: [w804 w812 w824 w835 w845 w855 w866 w877 w887 w896 w906 w920 w933 w941 w961 w974 w979 w988 w1001 w1009 w1024 w1045 w1056 w1063 w1075 w1087 w1106 w1117 w1124 w1133 w1142 w1151 w1163 w1168 w1179 w1189] -> w213
      tunnel: w207 -> [w799 _ _ _ _ _ _ _ _ _ _ _ _ _ _ _ _ _ _ _ _ _ _ _ _ _ w1099 _ _ _ _ _ _ _ _ _]
      tunnel: w206 -> [_ _ _ _ _ _ _ _ _ _ _ _ _ _ _ _ _ _ _ _ _ _ _ _ _ _ w1098 _ _ _ _ _ _ _ _ _]
      tunnel: w205 -> [w803 w811 w823 w834 w844 w854 w865 w876 w885 w893 w905 w919 w925 w938 w953 w971 w978 w987 w998 w1006 w1030 w1043 w1055 w1060 w1067 w1079 w1097 w1110 w1123 w1132 w1141 w1150 w1162 w1167 w1178 w1188]
      tunnel: [w803 w811 w823 w834 w844 w854 w865 w876 w885 w893 w905 w919 w925 w938 w952 w971 w978 w987 w998 w1006 w1029 w1043 w1055 w1060 w1067 w1079 w1091 w1110 w1123 w1132 w1141 w1150 w1162 w1167 w1178 w1188] -> w204
      tunnel: w202 -> [w802 w810 w822 w833 w843 w853 w864 w875 w884 w892 w904 w918 w934 w937 w958 w970 w977 w986 w997 w1005 w1020 w1042 w1052 w1059 w1066 w1078 w1090 w1109 w1120 w1129 w1138 w1147 w1159 w1169 w1180 w1190]
      tunnel: [w802 w810 w822 w833 w843 w853 w864 w875 w884 w892 w904 w918 w934 w937 w957 w970 w977 w986 w997 w1005 w1019 w1042 w1052 w1059 w1066 w1078 w1090 w1109 w1120 w1129 w1138 w1147 w1158 w1169 w1180 w1190] -> w201
      tunnel: w199 -> [w801 w809 w817 w828 w838 w852 w859 w870 w883 w891 w898 w911 w929 w936 w948 w969 w976 w985 w996 w1004 w1016 w1041 w1049 w1058 w1065 w1077 w1089 w1108 w1119 w1126 w1135 w1144 w1153 w1170 w1181 w1191]
      tunnel: [w801 w809 w817 w828 w838 w852 w859 w870 w883 w891 w898 w911 w928 w936 w947 w969 w976 w985 w996 w1004 w1015 w1041 w1049 w1058 w1065 w1077 w1089 w1108 w1119 w1126 w1135 w1144 w1153 w1170 w1181 w1191] -> w198
      tunnel: w196 -> [w798 w808 w818 w829 w839 w848 w860 w871 w880 w890 w897 w910 w924 w935 w942 w966 w975 w984 w995 w1002 w1013 w1039 w1048 w1057 w1064 w1076 w1088 w1107 w1118 w1125 w1134 w1143 w1152 w1164 w1174 w1184]
      tunnel: [w798 w808 w818 w829 w839 w848 w860 w871 w880 w890 w897 w910 w924 w935 w942 w966 w975 w984 w995 w1002 w1012 w1039 w1048 w1057 w1064 w1076 w1088 w1107 w1118 w1125 w1134 w1143 w1152 w1164 w1172 w1183] -> w195
      frame "Exit" {
        n60 = call "Imaq Dispose"("All Images? (No)"=TRUE, "Image"=w799) -> ()  [unwired: 4 in, 1 out]
      }
      frame "----Movement States----" {
      }
      frame "FORWARD" {
        # ">>> Time cluster >>>"
        # ">>> Yaw >>>"
        # ">>> Stepper position >>>"
        # ">>> Encoders >>>"
        # ">>> Object detection >>>"
        # ">>> Ultrasonic Sensors Detect >>>"
        n61 = Unbundle By Name(w817) -> ("Yaw"=w816:dbl)
        n62 = call "Motor Control NO PID AE Ver.vi"("Direction"=MOTOR_CONTROL_NO_PID_AE_DIRECTIONS_type_def."y-axis movement", "AE Mode"=MOTOR_CONTROL_NO_PID_AE_DATA_ENTRY_MODE_Type_def."Write to motors", "Speed"=0.5, "Yaw"=w816) -> ()  [unwired: 1 in, 2 out]
      }
      frame "LEFT" {
        n63 = Unbundle By Name(w828) -> ("Yaw"=w827:dbl)
        n64 = call "Motor Control NO PID AE Ver.vi"("Direction"=MOTOR_CONTROL_NO_PID_AE_DIRECTIONS_type_def."x-axis movement", "AE Mode"=MOTOR_CONTROL_NO_PID_AE_DATA_ENTRY_MODE_Type_def."Write to motors", "Speed"=-0.5, "Yaw"=w827) -> ()  [unwired: 1 in, 2 out]
      }
      frame "R-ACW" {
        n65 = call "Motor Control NO PID AE Ver.vi"("Direction"=MOTOR_CONTROL_NO_PID_AE_DIRECTIONS_type_def."Rotate", "AE Mode"=MOTOR_CONTROL_NO_PID_AE_DATA_ENTRY_MODE_Type_def."Write to motors", "Speed"=0.5) -> ()  [unwired: 2 in, 2 out]
      }
      frame "R-CW" {
        (unwired) -0.2 ("Speed")
        n66 = call "Motor Control NO PID AE Ver.vi"("Direction"=MOTOR_CONTROL_NO_PID_AE_DIRECTIONS_type_def."Rotate", "AE Mode"=MOTOR_CONTROL_NO_PID_AE_DATA_ENTRY_MODE_Type_def."Write to motors", "Speed"=-0.5) -> ()  [unwired: 2 in, 2 out]
      }
      frame "RIGHT" {
        n67 = Unbundle By Name(w859) -> ("Yaw"=w858:dbl)
        n68 = call "Motor Control NO PID AE Ver.vi"("Direction"=MOTOR_CONTROL_NO_PID_AE_DIRECTIONS_type_def."x-axis movement", "AE Mode"=MOTOR_CONTROL_NO_PID_AE_DATA_ENTRY_MODE_Type_def."Write to motors", "Speed"=-0.5, "Yaw"=w858) -> ()  [unwired: 1 in, 2 out]
      }
      frame "REVERSE" {
        n69 = Unbundle By Name(w870) -> ("Yaw"=w869:dbl)
        n70 = call "Motor Control NO PID AE Ver.vi"("Direction"=MOTOR_CONTROL_NO_PID_AE_DIRECTIONS_type_def."y-axis movement", "AE Mode"=MOTOR_CONTROL_NO_PID_AE_DATA_ENTRY_MODE_Type_def."Write to motors", "Speed"=-0.5, "Yaw"=w869) -> ()  [unwired: 1 in, 2 out]
      }
      frame "STOP" {
        n71 = Wait (ms)(milliseconds to wait=u32 500) -> ()  [unwired: 1 out]
        n72 = call "Motor Control NO PID AE Ver.vi"("Direction"=MOTOR_CONTROL_NO_PID_AE_DIRECTIONS_type_def."Stop", "AE Mode"=MOTOR_CONTROL_NO_PID_AE_DATA_ENTRY_MODE_Type_def."Write to motors") -> ()  [unwired: 3 in, 2 out]
      }
      frame "----SENSOR READING---- " {
      }
      frame "READ ENCODERS" {
        # ">>> Time cluster >>>"
        # ">>> Yaw >>>"
        # ">>> Stepper position >>>"
        # ">>> Object detection >>>"
        # ">>> Current encoder distance >>>"
        # ">>> Ultrasonic Sensors Detect >>>"
        n73 = call "Motor Control NO PID AE Ver.vi"("AE Mode"=MOTOR_CONTROL_NO_PID_AE_DATA_ENTRY_MODE_Type_def."Read from Encoders") -> ("Speed & distance"=w902:T1)  [unwired: 4 in, 1 out]
        n74 = Unbundle By Name(w902) -> ("xDistance"=w901:dbl, "yDistance"=w900:dbl, "wDistance"=w899:dbl)
        n75 = Bundle By Name(cluster=w907, "xDistance"=w901, "yDistance"=w900, "wDistance"=w899) -> (w906:T14)
      }
      frame "READ ULTRASONIC" {
        (unwired) navX_type_def."Read Values" ("Mode")
        (unwired) MOTOR_CONTROL_NO_PID_Type_Def."Latch" ("Direction")
        # ">>> Ultrasonic Sensors Detect >>>"
        # ">>> Object detection >>>"
        # ">>> Encoders >>>"
        # ">>> Stepper position >>>"
        # ">>> Yaw >>>"
        n76 = call "Arduino Interfacing VI.vi"("AE Mode"=Arduino_Interfacing."Read From Arduino") -> ("Arduino Data"=w916:T4)  [unwired: 3 in, 1 out]
        n77 = Unbundle By Name(w916) -> ("PING A"=w915:u8, "PING B"=w914:u8, "PING C"=w913:u8, "PING D"=w912:u8)
        n78 = Bundle By Name(cluster=w922, "PING_A"=w915, "PING_B"=w914, "PING_C"=w913, "PING_D"=w912) -> (w923:T13)
      }
      frame "READ YAW" {
        # ">>> Yaw >>>"
        # ">>> Ultrasonic Sensors Detect >>>"
        # ">>> Object detection >>>"
        # ">>> Encoders >>>"
        # ">>> Stepper position >>>"
        n79 = call "navX reading VI.vi"("Mode"=navX_type_def."Read Values") -> ("NavX Readings"=w927:T3)  [unwired: 2 in, 3 out]
        n80 = Unbundle By Name(w927) -> ("Yaw"=w926:dbl)
        n81 = Bundle By Name(cluster=w929, "Yaw"=w926) -> (w928:T9)
      }
      frame "----SYSTEM MODES----" {
        (unwired) I2C_MASTER_Type_Def."Last State" ("Arduino Mode")
        # ">>> Object detection >>>"
        # ">>> Yaw >>>"
        # ">>> Ultrasonic Sensors Detect >>>"
        # ">>> Encoders >>>"
        # ">>> Stepper position >>>"
      }
      frame "INIT" {
        w959 = u8 0
        w960 = 0.0
        # ">>> Object detection >>>"
        # ">>> Yaw >>>"
        # ">>> Ultrasonic Sensors Detect >>>"
        # ">>> Encoders >>>"
        # ">>> Stepper position >>>"
        # ">>State Logic  >>"
        n82 = call "Arduino Interfacing VI.vi"("AE Mode"=Arduino_Interfacing."Initialize") -> ()  [unwired: 3 in, 2 out]
        n83 = call "FGV Bool.vi"("Init/Read/Write State"=States_for_Action_Engine."Initialize") -> ()  [unwired: 2 in, 2 out]
        n84 = call "Motor Control NO PID AE Ver.vi"("AE Mode"=MOTOR_CONTROL_NO_PID_AE_DATA_ENTRY_MODE_Type_def."Initialize") -> ()  [unwired: 4 in, 2 out]
        n85 = call "Elasped Timer.vi"("Action"=Control."Initialize") -> ()  [unwired: 7 in, 4 out]
        n86 = Bundle By Name(cluster=w953, "Recognized Object"=FALSE, "Object X coordinate"=0.0, "Object Y coordinate"=0.0) -> (w952:T12)
        n87 = Bundle By Name(cluster=w958, "y Stepper Position"=u8 0, "z Stepper Position"=u8 0) -> (w957:T10)
        n88 = Bundle By Name(cluster=w962, "xDistance"=w960, "yDistance"=w960, "wDistance"=w960) -> (w961:T14)
        n89 = Bundle By Name(cluster=w964, "PING_A"=w959, "PING_B"=w959, "PING_C"=w959, "PING_D"=w959) -> (w965:T13)
        n90 = Bundle By Name(cluster=w948, "Yaw"=0.0) -> (w947:T9)
      }
      frame "ARDUINO - ULTRASONIC" {
        # ">>> Object detection >>>"
        # ">>> Yaw >>>"
        # ">>> Ultrasonic Sensors Detect >>>"
        # ">>> Encoders >>>"
        # ">>> Stepper position >>>"
        # ">>State Logic  >>"
        n91 = call "Arduino Interfacing VI.vi"("Data to Write"=I2C_MASTER_WRITE_NEW_Type_Def."Ultrasonic sensors", "AE Mode"=Arduino_Interfacing."Write to Arduino") -> ()  [unwired: 2 in, 2 out]
      }
      frame "NAVX CALIBRATE" {
        # ">>> Object detection >>>"
        # ">>> Yaw >>>"
        # ">>> Ultrasonic Sensors Detect >>>"
        # ">>> Encoders >>>"
        # ">>> Stepper position >>>"
        # ">>State Logic  >>"
        # "Adds a 15 second delay to the startup process \nfor the NavX to calibrate"
        n92 = Wait (ms)(milliseconds to wait=u32 5000) -> ()  [unwired: 1 out]
      }
      frame "NO ACTION", Default {
        (unwired) u8 0 ("y Stepper value")
        (unwired) TRUE ("Latch")
        (unwired) navX_type_def."Read Values" ("Mode")
        (unwired) MOTOR_CONTROL_NO_PID_Type_Def."Latch" ("Direction")
        # ">>> Object detection >>>"
        # ">>> Yaw >>>"
        # ">>> Ultrasonic Sensors Detect >>>"
        # ">>> Encoders >>>"
        # ">>> Stepper position >>>"
        # ">>State Logic  >>"
        n93 = case shown="4" w989 {
          tunnel: [0 100] -> w991
          frame 1, Default {
          }
          frame 4 {
          }
        }
      }
      frame "----RESET CASES----" {
        (unwired) I2C_MASTER_Type_Def."Last State" ("Arduino Mode")
        # ">>> Object detection >>>"
        # ">>> Yaw >>>"
        # ">>> Ultrasonic Sensors Detect >>>"
        # ">>> Encoders >>>"
        # ">>> Stepper position >>>"
        # ">>State Logic  >>"
      }
      frame "RESET ENCODERS" {
        # ">>> Object detection >>>"
        # ">>> Yaw >>>"
        # ">>> Ultrasonic Sensors Detect >>>"
        # ">>> Encoders >>>"
        # ">>> Stepper position >>>"
        # ">>State Logic  >>"
        n94 = call "Motor Control NO PID AE Ver.vi"("AE Mode"=MOTOR_CONTROL_NO_PID_AE_DATA_ENTRY_MODE_Type_def."Reset Encoders") -> ()  [unwired: 4 in, 2 out]
      }
      frame "RESET FLAGS" {
        (unwired) I2C_MASTER_Type_Def."Last State" ("Arduino Mode")
        # "Resets any software variables\nand/or non-critical states"
        n95 = Wait (ms)(milliseconds to wait=u32 20) -> ()  [unwired: 1 out]
        n96 = Bundle By Name(cluster=w1013, "Time up flag"=FALSE, "SET TIME TO CHECK"=0.0) -> (w1012:T8)
        n97 = Bundle By Name(cluster=w1030, "Recognized Object"=FALSE, "Object X coordinate"=0.0, "Object Y coordinate"=0.0) -> (w1029:T12)
        n98 = Bundle By Name(cluster=w1020, "y Stepper Position"=u8 0, "z Stepper Position"=u8 0) -> (w1019:T10)
        n99 = Bundle By Name(cluster=w1025, "xDistance"=0.0, "yDistance"=0.0, "wDistance"=0.0) -> (w1024:T14)
        n100 = Bundle By Name(cluster=w1037, "PING_A"=u8 0, "PING_B"=u8 0, "PING_C"=u8 0, "PING_D"=u8 0) -> (w1036:T13)
        n101 = Bundle By Name(cluster=w1016, "Yaw"=0.0) -> (w1015:T9)
      }
      frame "RESET YAW" {
        n102 = Wait (ms)(milliseconds to wait=u32 100) -> ()  [unwired: 1 out]
        n103 = call "navX reading VI.vi"("Mode"=navX_type_def."Zero Yaw") -> ()  [unwired: 2 in, 4 out]
      }
      frame "RESET ARM" {
        n104 = call "Arduino Interfacing VI.vi"("Data to Write"=I2C_MASTER_WRITE_NEW_Type_Def."Soft Reset", "AE Mode"=Arduino_Interfacing."Write to Arduino") -> ()  [unwired: 2 in, 2 out]
      }
      frame "--------CAM STATES-------" {
      }
      frame "OPEN LOG CAM" {
        n105 = call "Low-Level Grab.vi"("States"=State_control."Initialise", "Session In"=T29 "cam0") -> ("error out"=w1070:errorcluster, "Session Out"=w1071:T29)  [unwired: 7 in, 1 out]
        n106 = call "Low-Level Grab.vi"("error in (no error)"=w1070, "States"=State_control."Start camera", "Session In"=w1071) -> ()  [unwired: 6 in, 3 out]
      }
      frame "OPEN LIFE CAM" {
        (unwired) MOTOR_CONTROL_NO_PID_Type_Def."Latch" ("Direction")
        (unwired) navX_type_def."Read Values" ("Mode")
        n107 = call "Low-Level Grab.vi"("States"=State_control."Initialise", "Session In"=T29 "cam1") -> ("error out"=w1082:errorcluster, "Session Out"=w1083:T29)  [unwired: 7 in, 1 out]
        n108 = call "Low-Level Grab.vi"("error in (no error)"=w1082, "States"=State_control."Start camera", "Session In"=w1083) -> ()  [unwired: 6 in, 3 out]
      }
      frame "CAM ACQ" {
        # ">>> Yaw >>>"
        # ">>> Stepper position >>>"
        # ">>> Encoders >>>"
        # ">>> Object detection >>>"
        # ">>> Ultrasonic Sensors Detect >>>"
        # "Object detection"
        n109 = call "Low-Level Grab.vi"("error in (no error)"=w1098, "States"=State_control."Continuous Acquisition ") -> ("error out"=w1101:errorcluster, "Image Out"=w1102:T22)  [unwired: 7 in, 1 out]
        n110 = call "Object Detection SubVI.vi"("Error In"=w1101, "Mode"="Object recognition mode", "Image Dest"=w1099, "Image in"=w1102) -> ("Object Center Coordinates"=w1096:cluster{"x":sgl, "y":sgl}, "Object detection cluster"=w1093:T2)  [unwired: 2 out]
        "Object detection cluster" <- w1093
        "Object Center Coordinates" <- w1096
        n111 = Unbundle By Name(w1093) -> ("Object detected?"=w1092:bool)
        n112 = Unbundle By Name(w1096) -> ("x"=w1095:sgl, "y"=w1094:sgl)
        n113 = Bundle By Name(cluster=w1097, "Recognized Object"=w1092, "Object X coordinate"=w1095, "Object Y coordinate"=w1094) -> (w1091:T12)
      }
      frame "CAM CLOSE" {
        n114 = call "Low-Level Grab.vi"("States"=State_control."Stop camera") -> ("error out"=w1113:errorcluster, "Session Out"=w1114:T29)  [unwired: 8 in, 1 out]
        n115 = call "Low-Level Grab.vi"("error in (no error)"=w1113, "States"=State_control."Dispose all", "Session In"=w1114) -> ()  [unwired: 6 in, 3 out]
      }
      frame "-----ARM ACTIONS-----" {
      }
      frame "CLOSE CLAW" {
        n116 = call "Arduino Interfacing VI.vi"("Data to Write"=I2C_MASTER_WRITE_NEW_Type_Def."Close Claw", "AE Mode"=Arduino_Interfacing."Write to Arduino") -> ()  [unwired: 2 in, 2 out]
      }
      frame "OPEN CLAW" {
        n117 = call "Arduino Interfacing VI.vi"("Data to Write"=I2C_MASTER_WRITE_NEW_Type_Def."Open Claw", "AE Mode"=Arduino_Interfacing."Write to Arduino") -> ()  [unwired: 2 in, 2 out]
      }
      frame "Z STEPPER CAM HEIGHT" {
        n118 = call "Arduino Interfacing VI.vi"("Data to Write"=I2C_MASTER_WRITE_NEW_Type_Def."zStepper 8k", "AE Mode"=Arduino_Interfacing."Write to Arduino") -> ()  [unwired: 2 in, 2 out]
      }
      frame "READ STEPPER VALUES" {
        n119 = call "Arduino Interfacing VI.vi"("AE Mode"=Arduino_Interfacing."Read From Arduino") -> ("Arduino Data"=w1156:T4)  [unwired: 3 in, 1 out]
        n120 = Unbundle By Name(w1156) -> ("y Stepper Position"=w1155:u8, "z Stepper Position"=w1154:u8)
        n121 = Bundle By Name(cluster=w1159, "y Stepper Position"=w1155, "z Stepper Position"=w1154) -> (w1158:T10)
      }
      frame " -----TIMING-----" {
      }
      frame "SET TIMER" {
        n122 = call "Elasped Timer.vi"("Time Setting"=5.0, "Action"=Control."Initialize") -> ()  [unwired: 6 in, 4 out]
        n123 = Bundle By Name(cluster=w1174, "Time up flag"=FALSE) -> (w1172:T8)
      }
      frame "START TIMER" {
        n124 = call "Elasped Timer.vi"("Action"=Control."Start") -> ("Time Out?!"=w1182:bool)  [unwired: 7 in, 3 out]
        n125 = Bundle By Name(cluster=w1184, "Time up flag"=w1182) -> (w1183:T8)
      }
    }
    "State Logic" <- w217
    n126 = local read "TASK ENABLE"() -> (w211:bool)
    n127 = Not(x=w211) -> (.not. x?=w210:bool)
    n128 = case shown="True" w218 {
      tunnel: w222 -> [w244 w271]
      tunnel: w226 -> [w240 w273]
      tunnel: [w244 w271] -> w231
      tunnel: [w240 w274] -> w230
      tunnel: w227 -> [_ w269]
      tunnel: w229 -> [_ w270]
      tunnel: w224 -> [w243 w276]
      tunnel: [w243 w276] -> w223
      tunnel: "STOP TASK" -> [_ w259]
      tunnel: w217 -> [w242 w275]
      tunnel: [w242 w272] -> w216
      tunnel: w213 -> [w241 w265]
      tunnel: [w241 w265] -> w212
      tunnel: w210 -> [_ w260]
      tunnel: [w239 w257] -> w209
      tunnel: w208 -> [w239 w256]
      tunnel: w204 -> [w238 w253]
      tunnel: [w238 w253] -> w203
      tunnel: w201 -> [w237 w249]
      tunnel: [w237 w249] -> w200
      tunnel: w198 -> [w236 w247]
      tunnel: [w236 w247] -> w197
      tunnel: w195 -> [w235 w245]
      tunnel: [w235 w245] -> w194
      frame False {
        # ">>> Time cluster >>>"
        # ">>> Yaw >>>"
        # ">>> Stepper position >>>"
        # ">>> Encoders >>>"
        # ">>> Object detection >>>"
        # ">>> Ultrasonic Sensors Detect >>>"
      }
      frame True {
        # ">> Manual override >>"
        # ">>> Time cluster >>>"
        # ">>> Yaw >>>"
        # ">>> Stepper position >>>"
        # ">>> Encoders >>>"
        # ">>> Object detection >>>"
        # ">>> Ultrasonic Sensors Detect >>>"
        # ">>Action Queue>>"
        # ">>State Logic Queue Reference >>"
        n129 = Or(x=w259, y=w260) -> (x .or. y?=w258:bool)
        n130 = Unbundle By Name(w245) -> ("Time up flag"=w246:bool)
        "Time up flag" <- w246
        n131 = Unbundle By Name(w247) -> ("Yaw"=w248:dbl)
        n132 = Unbundle By Name(w249) -> ("y Stepper Position"=w251:u8, "z Stepper Position"=w250:u8)
        n133 = Unbundle By Name(w265) -> ("xDistance"=w262:dbl, "yDistance"=w263:dbl, "wDistance"=w264:dbl)
        n134 = Unbundle By Name(w253) -> ("Recognized Object"=w252:bool, "Object X coordinate"=w255:dbl, "Object Y coordinate"=w254:dbl)
        n135 = Unbundle By Name(w276) -> ("PING_A"=w268:u8, "PING_B"=w267:u8, "PING_C"=w266:u8, "PING_D"=w261:u8)
        n136 = case shown="23" w275 {
          tunnel: [w278 w281 w292 w299 w358 w370 w406 w452 w496 w553 w590 w644 w684 w728 w769] -> w274
          tunnel: w273 -> [w278 w284 w293 w302 w360 w371 w407 w453 w502 w546 w594 w634 w687 w723 w760]
          tunnel: [State_Type_Definitions,_for_0.26g_versions_and_later_2."Idle" ("Enum") State_Type_Definitions,_for_0.26g_versions_and_later_2."Idle" ("Enum") w288 w301 State_Type_Definitions,_for_0.26g_versions_and_later_2."Shutdown" ("Enum") w372 w409 w451 w497 w552 w591 w643 w685 w729 w761] -> w272
          tunnel: w271 -> [_ _ w291 w305 _ w377 w419 w460 w501 w550 w595 w641 w679 w726 w768]
          tunnel: w270 -> [_ _ _ w304 _ w376 w418 w459 w500 w549 w587 w640 w678 w725 w766]
          tunnel: w269 -> [_ _ w290 w300 _ w375 w417 w458 w499 w548 w586 w642 w680 w724 w767]
          tunnel: w258 -> [_ _ _ _ _ w369 w408 w455 w495 w551 w592 w635 w688 w727 w764]
          tunnel: w268 -> [_ _ _ _ _ _ _ _ _ _ _ _ _ _ _]
          tunnel: w267 -> [_ _ _ _ _ _ w415 _ w493 w541 w597 _ _ _ _]
          tunnel: w266 -> [_ _ _ _ _ _ w414 _ w494 w542 w596 _ _ _ _]
          tunnel: w264 -> [_ _ _ _ _ _ _ w457 _ _ _ _ _ _ _]
          tunnel: w263 -> [_ _ _ _ _ w368 _ _ _ _ _ _ _ _ _]
          tunnel: w262 -> [_ _ _ _ _ _ _ _ _ w537 _ _ _ _ _]
          tunnel: w261 -> [_ _ _ _ _ _ _ _ _ _ _ _ _ _ _]
          tunnel: [State_Type_Definitions,_for_0.26g_versions_and_later_2."Idle" ("Enum") State_Type_Definitions,_for_0.26g_versions_and_later_2."Idle" ("Enum") State_Type_Definitions,_for_0.26g_versions_and_later_2."Idle" ("Enum") State_Type_Definitions,_for_0.26g_versions_and_later_2."Idle" ("Enum") State_Type_Definitions,_for_0.26g_versions_and_later_2."Shutdown" ("Enum") w365 w405 w448 w488 w536 w589 w645 w686 w730 w762] -> w257
          tunnel: w256 -> [_ _ w288 _ _ _ _ _ _ _ _ _ _ _ _]
          tunnel: w252 -> [_ _ _ _ _ _ _ _ _ _ _ _ w683 _ w763]
          tunnel: w255 -> [_ _ _ _ _ _ _ _ _ _ _ _ _ _ _]
          tunnel: w254 -> [_ _ _ _ _ _ _ _ _ _ _ _ _ _ _]
          tunnel: w251 -> [_ _ _ _ _ _ _ _ _ _ _ _ _ _ _]
          tunnel: w250 -> [_ _ _ _ _ _ _ _ _ _ _ w638 _ w722 _]
          tunnel: w248 -> [_ _ _ _ _ _ _ _ _ _ _ _ _ _ _]
          tunnel: w246 -> [_ _ _ _ _ _ _ _ _ _ _ _ w682 _ _]
          frame 0 {
          }
          frame 1 {
            n137 = for {
              shift-right: [w287] -> w281
              shift-left: w284 -> [w286]
              tunnel: string[] ["INIT", "RESET ARM", "RESET FLAGS", "RESET YAW", "NAVX CALIBRATE"] -> [w285] mode=indexing
              n138 = Enqueue Element(queue=w286, element=w285) -> (queue out=w287:refnum<queue>)  [unwired: 2 in, 2 out]
            }
          }
          frame 3 {
            n139 = Flush Queue(queue=w291, error in (no error)=w290) -> ()  [unwired: 3 out]
            n140 = for {
              shift-right: [w297] -> w292
              shift-left: w293 -> [w296]
              tunnel: string[] ["STOP", "RESET ENCODERS", "RESET YAW", "ARDUINO MODE 0", "CAM CLOSE", "RESET ARM"] -> [w295] mode=indexing
              n141 = Enqueue Element(queue=w296, element=w295) -> (queue out=w297:refnum<queue>)  [unwired: 2 in, 2 out]
            }
          }
          frame 4, Default {
            (unwired) TRUE ("Green LED")
            n142 = Dequeue Element(queue=w305, timeout in ms (-1)=w304, error in (no error)=w300) -> (element=w303:T7)  [unwired: 3 out]
            n143 = case shown="\"Start Task 5\"" w303 {
              tunnel: [w307 w314 w321 w328 w335 w342 w349 w351] -> w299
              tunnel: w302 -> [w308 w315 w322 w329 w336 w343 w349 w352]
              tunnel: [State_Type_Definitions."Task 1" ("Enum") State_Type_Definitions."Task 2" ("Enum") State_Type_Definitions,_for_0.26g_versions_and_later_2."Task 3" ("Enum") State_Type_Definitions,_for_0.26g_versions_and_later_2."Task 4_A" ("Enum") State_Type_Definitions."Task 5_A" ("Enum") State_Type_Definitions,_for_0.26g_versions_and_later_2."Task 6_A" ("Enum") State_Type_Definitions,_for_0.26g_versions_and_later_2."Idle" ("Enum") State_Type_Definitions,_for_0.26g_versions_and_later_2."Shutdown" ("Enum")] -> w301
              frame "Start Task 1" {
                n144 = for {
                  shift-right: [w312] -> w307
                  shift-left: w308 -> [w311]
                  tunnel: string[] ["RESET ENCODERS", "RESET YAW", "FORWARD", "READ ENCODERS"] -> [w310] mode=indexing
                  n145 = Enqueue Element(queue=w311, element=w310) -> (queue out=w312:refnum<queue>)  [unwired: 2 in, 2 out]
                }
              }
              frame "Start Task 2" {
                n146 = for {
                  shift-right: [w319] -> w314
                  shift-left: w315 -> [w318]
                  tunnel: string[] ["RESET ENCODERS", "RESET YAW", "READ ULTRASONIC", "ARDUINO - ULTRASONIC"] -> [w317] mode=indexing
                  n147 = Enqueue Element(queue=w318, element=w317) -> (queue out=w319:refnum<queue>)  [unwired: 2 in, 2 out]
                }
              }
              frame "Start Task 3" {
                n148 = for {
                  shift-right: [w326] -> w321
                  shift-left: w322 -> [w325]
                  tunnel: string[] ["RESET ENCODERS", "READ ENCODERS", "R-ACW"] -> [w324] mode=indexing
                  n149 = Enqueue Element(queue=w325, element=w324) -> (queue out=w326:refnum<queue>)  [unwired: 2 in, 2 out]
                }
              }
              frame "Start Task 4" {
                n150 = for {
                  shift-right: [w333] -> w328
                  shift-left: w329 -> [w332]
                  tunnel: string[] ["STOP", "RESET YAW", "RESET ENCODERS", "READ ULTRASONIC", "ARDUINO - ULTRASONIC", ""] -> [w331] mode=indexing
                  n151 = Enqueue Element(queue=w332, element=w331) -> (queue out=w333:refnum<queue>)  [unwired: 2 in, 2 out]
                }
              }
              frame "Start Task 5" {
                n152 = for {
                  shift-right: [w340] -> w335
                  shift-left: w336 -> [w339]
                  tunnel: string[] ["RESET YAW", "RESET ENCODERS", "READ STEPPER VALUES", "Z STEPPER CAM HEIGHT", "", ""] -> [w338] mode=indexing
                  n153 = Enqueue Element(queue=w339, element=w338) -> (queue out=w340:refnum<queue>)  [unwired: 2 in, 2 out]
                }
              }
              frame "Start Task 6" {
                n154 = for {
                  shift-right: [w347] -> w342
                  shift-left: w343 -> [w346]
                  tunnel: string[] ["Z STEPPER CAM HEIGHT ", "READ STEPPER VALUES", "OPEN LOG CAM", "", "", ""] -> [w345] mode=indexing
                  n155 = Enqueue Element(queue=w346, element=w345) -> (queue out=w347:refnum<queue>)  [unwired: 2 in, 2 out]
                }
              }
              frame "None", Default {
              }
              frame "Exit" {
                n156 = for {
                  shift-right: [w356] -> w351
                  shift-left: w352 -> [w355]
                  tunnel: string[] ["STOP", "RESET ENCODERS", "RESET YAW", "EXIT"] -> [w354] mode=indexing
                  n157 = Enqueue Element(queue=w355, element=w354) -> (queue out=w356:refnum<queue>)  [unwired: 2 in, 2 out]
                }
              }
            }
          }
          frame 5 {
            n158 = for {
              shift-right: [w364] -> w358
              shift-left: w360 -> [w363]
              tunnel: string[] ["INIT", "RESET ENCODERS", "RESET FLAGS", "EXIT"] -> [w362] mode=indexing
              n159 = Enqueue Element(queue=w363, element=w362) -> (queue out=w364:refnum<queue>)  [unwired: 2 in, 2 out]
            }
          }
          frame 6 {
            # "Use 250"
            n160 = Dequeue Element(queue=w377, timeout in ms (-1)=w376, error in (no error)=w375) -> (element=w374:T7)  [unwired: 3 out]
            n161 = Greater?(x=w368, y=10000.0) -> (0:w366:bool)
            n162 = Or(x=w366, y=w369) -> (x .or. y?=w373:bool)
            n163 = case shown="\"None\", Default" w374 {
              tunnel: w373 -> [w380 _]
              tunnel: [w384 State_Type_Definitions,_for_0.26g_versions_and_later_2."True Stop" ("Enum")] -> w372
              tunnel: w371 -> [w381 w399]
              tunnel: [w379 w398] -> w370
              tunnel: [State_Type_Definitions,_for_0.26g_versions_and_later_2."Idle" ("Enum") State_Type_Definitions,_for_0.26g_versions_and_later_2."Shutdown" ("Enum")] -> w365
              frame "None", Default {
                n164 = case shown="True" w380 {
                  tunnel: w381 -> [w387 w393]
                  tunnel: [w386 w391] -> w379
                  frame False {
                    n165 = for {
                      shift-right: [w389] -> w386
                      shift-left: w387 -> [w390]
                      tunnel: string[] ["READ ENCODERS", "READ YAW", "FORWARD"] ("element") -> [w388] mode=indexing
                      n166 = Enqueue Element(queue=w390, element=w388) -> (queue out=w389:refnum<queue>)  [unwired: 2 in, 2 out]
                    }
                  }
                  frame True {
                    n167 = for {
                      shift-right: [w395] -> w391
                      shift-left: w393 -> [w396]
                      tunnel: string[] ["RESET YAW", "RESET ENCODERS", "STOP", ""] -> [w394] mode=indexing
                      n168 = Enqueue Element(queue=w396, element=w394) -> (queue out=w395:refnum<queue>)  [unwired: 2 in, 2 out]
                    }
                  }
                }
                n169 = Select(t=State_Type_Definitions,_for_0.26g_versions_and_later_2."True Stop" ("Enum"), s=w380, f=State_Type_Definitions."Task 1" ("Enum")) -> (s? t:f=w384:u16)
              }
              frame "Exit" {
                n170 = for {
                  shift-right: [w403] -> w398
                  shift-left: w399 -> [w404]
                  tunnel: string[] ["STOP", "RESET ENCODERS", "RESET YAW", ""] -> [w402] mode=indexing
                  n171 = Enqueue Element(queue=w404, element=w402) -> (queue out=w403:refnum<queue>)  [unwired: 2 in, 2 out]
                }
              }
            }
          }
          frame 7 {
            w413 = u8 10 ("y")
            # ">>Object detected>>"
            n172 = Dequeue Element(queue=w419, timeout in ms (-1)=w418, error in (no error)=w417) -> (element=w416:T7)  [unwired: 3 out]
            n173 = Less?(x=w415, y=w413) -> (x < y?=w412:bool)
            n174 = Less?(x=w414, y=w413) -> (x < y?=w411:bool)
            n175 = Or(x=w412, y=w411) -> (x .or. y?=w410:bool)
            "Object detected?" <- w410
            n176 = case shown="\"None\", Default" w416 {
              tunnel: w410 -> [w423 _]
              tunnel: [w425 State_Type_Definitions,_for_0.26g_versions_and_later_2."True Stop" ("Enum")] -> w409
              tunnel: w408 -> [w424 _]
              tunnel: w407 -> [w422 w442]
              tunnel: [w421 w443] -> w406
              tunnel: [State_Type_Definitions,_for_0.26g_versions_and_later_2."Idle" ("Enum") State_Type_Definitions,_for_0.26g_versions_and_later_2."Shutdown" ("Enum")] -> w405
              frame "None", Default {
                n177 = case shown="False" w423 {
                  tunnel: w422 -> [w429 w436]
                  tunnel: [w430 w435] -> w421
                  frame False {
                    n178 = for {
                      tunnel: string[] ["READ ULTRASONIC", "STOP"] ("element") -> [w431] mode=indexing
                      shift-right: [w433] -> w430
                      shift-left: w429 -> [w432]
                      n179 = Enqueue Element(queue=w432, element=w431) -> (queue out=w433:refnum<queue>)  [unwired: 2 in, 2 out]
                    }
                  }
                  frame True {
                    n180 = for {
                      shift-right: [w438] -> w435
                      shift-left: w436 -> [w439]
                      tunnel: string[] ["REVERSE", "READ ULTRASONIC"] -> [w437] mode=indexing
                      n181 = Enqueue Element(queue=w439, element=w437) -> (queue out=w438:refnum<queue>)  [unwired: 2 in, 2 out]
                    }
                  }
                }
                n182 = Select(t=State_Type_Definitions,_for_0.26g_versions_and_later_2."True Stop" ("Enum"), s=w424, f=State_Type_Definitions."Task 2" ("Enum")) -> (s? t:f=w425:u16)
              }
              frame "Exit" {
                n183 = for {
                  shift-right: [w446] -> w443
                  shift-left: w442 -> [w447]
                  tunnel: string[] ["STOP", "RESET ENCODERS", "RESET YAW", "ARDUINO MODE 0"] -> [w445] mode=indexing
                  n184 = Enqueue Element(queue=w447, element=w445) -> (queue out=w446:refnum<queue>)  [unwired: 2 in, 2 out]
                }
              }
            }
          }
          frame 10 {
            n185 = Dequeue Element(queue=w460, timeout in ms (-1)=w459, error in (no error)=w458) -> (element=w449:T7)  [unwired: 3 out]
            n186 = Greater?(x=w457, y=150.0) -> (0:w454:bool)
            n187 = Or(x=w454, y=w455) -> (x .or. y?=w450:bool)
            n188 = case shown="\"Exit\"" w449 {
              tunnel: w450 -> [w463 _]
              tunnel: [w467 State_Type_Definitions,_for_0.26g_versions_and_later_2."True Stop" ("Enum")] -> w451
              tunnel: w453 -> [w464 w483]
              tunnel: [w462 w482] -> w452
              tunnel: [State_Type_Definitions,_for_0.26g_versions_and_later_2."Idle" ("Enum") State_Type_Definitions,_for_0.26g_versions_and_later_2."Shutdown" ("Enum")] -> w448
              frame "None", Default {
                n189 = case shown="False" w463 {
                  tunnel: w464 -> [w470 w476]
                  tunnel: [w469 w474] -> w462
                  frame False {
                    n190 = for {
                      shift-right: [w472] -> w469
                      shift-left: w470 -> [w473]
                      tunnel: string[] ["READ ENCODERS", "R-ACW"] ("element") -> [w471] mode=indexing
                      n191 = Enqueue Element(queue=w473, element=w471) -> (queue out=w472:refnum<queue>)  [unwired: 2 in, 2 out]
                    }
                  }
                  frame True {
                    n192 = for {
                      shift-right: [w478] -> w474
                      shift-left: w476 -> [w479]
                      tunnel: string[] ["RESET YAW", "RESET ENCODERS", "STOP", "ARDUINO MODE 0"] -> [w477] mode=indexing
                      n193 = Enqueue Element(queue=w479, element=w477) -> (queue out=w478:refnum<queue>)  [unwired: 2 in, 2 out]
                    }
                  }
                }
                n194 = Select(t=State_Type_Definitions,_for_0.26g_versions_and_later_2."True Stop" ("Enum"), s=w463, f=State_Type_Definitions,_for_0.26g_versions_and_later_2."Task 3" ("Enum")) -> (s? t:f=w467:T6)
              }
              frame "Exit" {
                n195 = for {
                  shift-right: [w486] -> w482
                  shift-left: w483 -> [w487]
                  tunnel: string[] ["STOP", "RESET ENCODERS", "RESET YAW", ""] -> [w485] mode=indexing
                  n196 = Enqueue Element(queue=w487, element=w485) -> (queue out=w486:refnum<queue>)  [unwired: 2 in, 2 out]
                }
              }
            }
          }
          frame 11 {
            w492 = 20
            # ">> Outputs true if object detected >>"
            # ">> Manual override >>"
            n197 = Dequeue Element(queue=w501, timeout in ms (-1)=w500, error in (no error)=w499) -> (element=w498:T7)  [unwired: 3 out]
            n198 = Less?(x=w494, y=w492) -> (x < y?=w490:bool)
            n199 = Less?(x=w493, y=w492) -> (x < y?=w491:bool)
            n200 = And(x=w491, y=w490) -> (x .and. y?=w489:bool)
            "Detect?" <- w489
            n201 = case shown="\"None\", Default" w498 {
              tunnel: [w511 State_Type_Definitions,_for_0.26g_versions_and_later_2."True Stop" ("Enum")] -> w497
              tunnel: [w509 w530] -> w496
              tunnel: w502 -> [w508 _]
              tunnel: w495 -> [w506 _]
              tunnel: w489 -> [w504 _]
              tunnel: [w503 State_Type_Definitions,_for_0.26g_versions_and_later_2."Shutdown" ("Enum")] -> w488
              frame "None", Default {
                # ">> WIill proceed to part ii if not manual override >>"
                # ">>If ENABLE or Trigger is set to true>>"
                n202 = Or(x=w504, y=w506) -> (x .or. y?=w505:bool)
                n203 = case shown="False" w505 {
                  tunnel: [w518 w523] -> w509
                  tunnel: w508 -> [w516 w522]
                  frame False {
                    n204 = for {
                      shift-right: [w520] -> w518
                      shift-left: w516 -> [w521]
                      tunnel: string[] ["FORWARD", "ULTRASONIC READ", ""] ("element") -> [w519] mode=indexing
                      n205 = Enqueue Element(queue=w521, element=w519) -> (queue out=w520:refnum<queue>)  [unwired: 2 in, 2 out]
                    }
                  }
                  frame True {
                    n206 = for {
                      shift-right: [w526] -> w523
                      shift-left: w522 -> [w527]
                      tunnel: string[] ["STOP", "RESET ENCODERS", "RESET YAW", "ARDUINO MODE 0"] -> [w525] mode=indexing
                      n207 = Enqueue Element(queue=w527, element=w525) -> (queue out=w526:refnum<queue>)  [unwired: 2 in, 2 out]
                    }
                  }
                }
                n208 = case shown="False" w506 {
                  tunnel: [State_Type_Definitions,_for_0.26g_versions_and_later_2."True Stop" ("Enum") State_Type_Definitions,_for_0.26g_versions_and_later_2."True Stop" ("Enum")] -> w507
                  tunnel: [State_Type_Definitions,_for_0.26g_versions_and_later_2."Task 4_B" ("Enum") State_Type_Definitions,_for_0.26g_versions_and_later_2."Idle" ("Enum")] -> w503
                  frame False {
                  }
                  frame True {
                  }
                }
                n209 = Select(t=w507, s=w505, f=State_Type_Definitions,_for_0.26g_versions_and_later_2."Task 4_A" ("Enum")) -> (s? t:f=w511:T6)
              }
              frame "Exit" {
                n210 = for {
                  shift-right: [w533] -> w530
                  shift-left: _ -> [w534]
                  tunnel: string[] ["STOP", "RESET ENCODERS", "RESET YAW", ""] -> [w532] mode=indexing
                  n211 = Enqueue Element(queue=w534, element=w532) -> (queue out=w533:refnum<queue>)  [unwired: 2 in, 2 out]
                }
              }
            }
          }
          frame 12 {
            w545 = 20
            # ">> Outputs true if 150 mm has been moved >>"
            # ">> Outputs true if sensor not obstructed>>"
            # ">> Manual override >>"
            n212 = Dequeue Element(queue=w550, timeout in ms (-1)=w549, error in (no error)=w548) -> (element=w547:T7)  [unwired: 3 out]
            n213 = Greater?(x=w542, y=w545) -> (0:w543:bool)
            n214 = Greater?(x=w541, y=w545) -> (0:w544:bool)
            n215 = Greater Or Equal?(x=w537, y=80.0) -> (x >= y?=w539:bool)
            n216 = And(x=w544, y=w543) -> (x .and. y?=w538:bool)
            n217 = And(x=w539, y=w538) -> (x .and. y?=w535:bool)
            n218 = case shown="\"None\", Default" w547 {
              tunnel: [w562 State_Type_Definitions,_for_0.26g_versions_and_later_2."True Stop" ("Enum")] -> w552
              tunnel: [w560 w581] -> w553
              tunnel: w546 -> [w559 _]
              tunnel: w551 -> [w557 _]
              tunnel: w535 -> [w555 _]
              tunnel: [w554 State_Type_Definitions,_for_0.26g_versions_and_later_2."Shutdown" ("Enum")] -> w536
              frame "None", Default {
                # ">> WIill proceed to part ii if not manual override >>"
                # ">>If ENABLE or Trigger is set to true>>"
                n219 = Or(x=w555, y=w557) -> (x .or. y?=w556:bool)
                n220 = case shown="False" w556 {
                  tunnel: [w569 w574] -> w560
                  tunnel: w559 -> [w567 w573]
                  frame False {
                    n221 = for {
                      shift-right: [w571] -> w569
                      shift-left: w567 -> [w572]
                      tunnel: string[] ["RIGHT", "ULTRASONIC READ", "READ ENCODERS"] ("element") -> [w570] mode=indexing
                      n222 = Enqueue Element(queue=w572, element=w570) -> (queue out=w571:refnum<queue>)  [unwired: 2 in, 2 out]
                    }
                  }
                  frame True {
                    n223 = for {
                      shift-right: [w577] -> w574
                      shift-left: w573 -> [w578]
                      tunnel: string[] ["STOP", "RESET ENCODERS", "RESET YAW", "ARDUINO MODE 0"] -> [w576] mode=indexing
                      n224 = Enqueue Element(queue=w578, element=w576) -> (queue out=w577:refnum<queue>)  [unwired: 2 in, 2 out]
                    }
                  }
                }
                n225 = case shown="True" w557 {
                  tunnel: [State_Type_Definitions,_for_0.26g_versions_and_later_2."True Stop" ("Enum") State_Type_Definitions,_for_0.26g_versions_and_later_2."True Stop" ("Enum")] -> w558
                  tunnel: [State_Type_Definitions,_for_0.26g_versions_and_later_2."Task 4_C" ("Enum") State_Type_Definitions,_for_0.26g_versions_and_later_2."Idle" ("Enum")] -> w554
                  frame False {
                  }
                  frame True {
                  }
                }
                n226 = Select(t=w558, s=w556, f=State_Type_Definitions,_for_0.26g_versions_and_later_2."Task 4_B" ("Enum")) -> (s? t:f=w562:T6)
              }
              frame "Exit" {
                n227 = for {
                  shift-right: [w584] -> w581
                  shift-left: _ -> [w585]
                  tunnel: string[] ["STOP", "RESET ENCODERS", "RESET YAW", ""] -> [w583] mode=indexing
                  n228 = Enqueue Element(queue=w585, element=w583) -> (queue out=w584:refnum<queue>)  [unwired: 2 in, 2 out]
                }
              }
            }
          }
          frame 13 {
            w600 = u8 20
            # ">> Outputs true if object detected >>"
            # ">> Manual override >>"
            n229 = Dequeue Element(queue=w595, timeout in ms (-1)=w587, error in (no error)=w586) -> (element=w588:T7)  [unwired: 3 out]
            n230 = Less?(x=w596, y=w600) -> (x < y?=w598:bool)
            n231 = Less?(x=w597, y=w600) -> (x < y?=w599:bool)
            n232 = And(x=w599, y=w598) -> (x .and. y?=w593:bool)
            n233 = case shown="\"None\", Default" w588 {
              tunnel: [w609 State_Type_Definitions,_for_0.26g_versions_and_later_2."True Stop" ("Enum")] -> w591
              tunnel: [w607 w629] -> w590
              tunnel: w594 -> [w606 w626]
              tunnel: w592 -> [w604 _]
              tunnel: w593 -> [w602 _]
              tunnel: [w601 State_Type_Definitions,_for_0.26g_versions_and_later_2."Shutdown" ("Enum")] -> w589
              frame "None", Default {
                # ">> WIill proceed to part ii if not manual override >>"
                # ">>If ENABLE or Trigger is set to true>>"
                n234 = Or(x=w602, y=w604) -> (x .or. y?=w603:bool)
                n235 = case shown="False" w603 {
                  tunnel: [w616 w621] -> w607
                  tunnel: w606 -> [w614 w620]
                  frame False {
                    n236 = for {
                      shift-right: [w618] -> w616
                      shift-left: w614 -> [w619]
                      tunnel: string[] ["FORWARD", "ULTRASONIC READ", ""] ("element") -> [w617] mode=indexing
                      n237 = Enqueue Element(queue=w619, element=w617) -> (queue out=w618:refnum<queue>)  [unwired: 2 in, 2 out]
                    }
                  }
                  frame True {
                    n238 = for {
                      shift-right: [w624] -> w621
                      shift-left: w620 -> [w625]
                      tunnel: string[] ["STOP", "RESET ENCODERS", "RESET YAW", "ARDUINO MODE 0"] -> [w623] mode=indexing
                      n239 = Enqueue Element(queue=w625, element=w623) -> (queue out=w624:refnum<queue>)  [unwired: 2 in, 2 out]
                    }
                  }
                }
                n240 = case shown="True" w604 {
                  tunnel: [State_Type_Definitions,_for_0.26g_versions_and_later_2."True Stop" ("Enum") State_Type_Definitions,_for_0.26g_versions_and_later_2."True Stop" ("Enum")] -> w605
                  tunnel: [State_Type_Definitions,_for_0.26g_versions_and_later_2."Idle" ("Enum") State_Type_Definitions,_for_0.26g_versions_and_later_2."Idle" ("Enum")] -> w601
                  frame False {
                  }
                  frame True {
                  }
                }
                n241 = Select(t=w605, s=w603, f=State_Type_Definitions,_for_0.26g_versions_and_later_2."Task 4_C" ("Enum")) -> (s? t:f=w609:T6)
              }
              frame "Exit" {
                n242 = for {
                  shift-right: [w632] -> w629
                  shift-left: w626 -> [w633]
                  tunnel: string[] ["STOP", "RESET ENCODERS", "RESET YAW", ""] -> [w631] mode=indexing
                  n243 = Enqueue Element(queue=w633, element=w631) -> (queue out=w632:refnum<queue>)  [unwired: 2 in, 2 out]
                }
              }
            }
          }
          frame 12 {
            # ">> Manual override >>"
            n244 = Dequeue Element(queue=w641, timeout in ms (-1)=w640, error in (no error)=w642) -> (element=w639:T7)  [unwired: 3 out]
            n245 = Equal?(x=w638, y=u8 80) -> (x = y?=w636:bool)
            n246 = case shown="\"None\", Default" w639 {
              tunnel: [w652 State_Type_Definitions,_for_0.26g_versions_and_later_2."True Stop" ("Enum")] -> w643
              tunnel: [w655 w672] -> w644
              tunnel: [State_Type_Definitions,_for_0.26g_versions_and_later_2."Idle" ("Enum") State_Type_Definitions,_for_0.26g_versions_and_later_2."Shutdown" ("Enum")] -> w645
              tunnel: w636 -> [w651 _]
              tunnel: w635 -> [w650 _]
              tunnel: w634 -> [w646 w669]
              frame "None", Default {
                # "Stays in Task 5_A until stepper reaches desired \nheight"
                # "T: Go back to idle, F: Continue with task\""
                # ">> Manual override >>"
                n247 = case shown="True" w651 {
                  tunnel: [w659 w665] -> w655
                  tunnel: w646 -> [w657 w663]
                  frame False {
                    n248 = for {
                      tunnel: string[] ["Z STEPPER CAM HEIGHT", "READ STEPPER VALUES"] ("element") -> [w660] mode=indexing
                      shift-right: [w662] -> w659
                      shift-left: w657 -> [w661]
                      n249 = Enqueue Element(queue=w661, element=w660) -> (queue out=w662:refnum<queue>)  [unwired: 2 in, 2 out]
                    }
                  }
                  frame True {
                    n250 = for {
                      shift-right: [w667] -> w665
                      shift-left: w663 -> [w668]
                      tunnel: string[] ["OPEN LOG CAM", "SET TIMER", ""] -> [w666] mode=indexing
                      n251 = Enqueue Element(queue=w668, element=w666) -> (queue out=w667:refnum<queue>)  [unwired: 2 in, 2 out]
                    }
                  }
                }
                n252 = Or(x=w651, y=w650) -> (x .or. y?=w653:bool)
                n253 = Select(t=State_Type_Definitions,_for_0.26g_versions_and_later_2."True Stop" ("Enum"), s=w650, f=State_Type_Definitions."Task 5 _B" ("Enum")) -> (s? t:f=w647:u16)
                n254 = Select(t=w647, s=w653, f=State_Type_Definitions."Task 5_A" ("Enum")) -> (s? t:f=w652:u16)
              }
              frame "Exit" {
                n255 = for {
                  shift-right: [w675] -> w672
                  shift-left: w669 -> [w676]
                  tunnel: string[] ["STOP", "RESET ENCODERS", "RESET YAW", "ARDUINO MODE 0"] -> [w674] mode=indexing
                  n256 = Enqueue Element(queue=w676, element=w674) -> (queue out=w675:refnum<queue>)  [unwired: 2 in, 2 out]
                }
              }
            }
          }
          frame 13 {
            n257 = Dequeue Element(queue=w679, timeout in ms (-1)=w678, error in (no error)=w680) -> (element=w677:T7)  [unwired: 3 out]
            n258 = And(x=w682, y=w683) -> (x .and. y?=w681:bool)
            "Recognized object + Time up?" <- w681
            n259 = case shown="\"None\", Default" w677 {
              tunnel: [w695 State_Type_Definitions,_for_0.26g_versions_and_later_2."True Stop" ("Enum")] -> w685
              tunnel: [w698 w715] -> w684
              tunnel: [State_Type_Definitions,_for_0.26g_versions_and_later_2."Idle" ("Enum") State_Type_Definitions,_for_0.26g_versions_and_later_2."Shutdown" ("Enum")] -> w686
              tunnel: w681 -> [w694 _]
              tunnel: w688 -> [w693 _]
              tunnel: w687 -> [w689 w712]
              frame "None", Default {
                # "Stays in Task 5_B until time is up and object is detected"
                # "T: Go back to idle, F: Continue with task\""
                # ">> Manual override >>"
                n260 = case shown="False" w694 {
                  tunnel: [w702 w708] -> w698
                  tunnel: w689 -> [w700 w706]
                  frame False {
                    n261 = for {
                      tunnel: string[] ["CAM ACQ", "START TIMER"] ("element") -> [w703] mode=indexing
                      shift-right: [w705] -> w702
                      shift-left: w700 -> [w704]
                      n262 = Enqueue Element(queue=w704, element=w703) -> (queue out=w705:refnum<queue>)  [unwired: 2 in, 2 out]
                    }
                  }
                  frame True {
                    n263 = for {
                      shift-right: [w710] -> w708
                      shift-left: w706 -> [w711]
                      tunnel: string[] ["CAM CLOSE", "SET TIMER"] -> [w709] mode=indexing
                      n264 = Enqueue Element(queue=w711, element=w709) -> (queue out=w710:refnum<queue>)  [unwired: 2 in, 2 out]
                    }
                  }
                }
                n265 = Or(x=w694, y=w693) -> (x .or. y?=w696:bool)
                n266 = Select(t=State_Type_Definitions,_for_0.26g_versions_and_later_2."True Stop" ("Enum"), s=w693, f=State_Type_Definitions,_for_0.26g_versions_and_later_2."True Stop" ("Enum")) -> (s? t:f=w690:T6)
                n267 = Select(t=w690, s=w696, f=State_Type_Definitions."Task 5 _B" ("Enum")) -> (s? t:f=w695:u16)
              }
              frame "Exit" {
                n268 = for {
                  shift-right: [w718] -> w715
                  shift-left: w712 -> [w719]
                  tunnel: string[] ["STOP", "RESET ENCODERS", "RESET YAW", "ARDUINO MODE 0"] -> [w717] mode=indexing
                  n269 = Enqueue Element(queue=w719, element=w717) -> (queue out=w718:refnum<queue>)  [unwired: 2 in, 2 out]
                }
              }
            }
          }
          frame 23 {
            n270 = Dequeue Element(queue=w726, timeout in ms (-1)=w725, error in (no error)=w724) -> (element=w731:T7)  [unwired: 3 out]
            n271 = Equal?(x=w722, y=u8 80) -> (x = y?=w721:bool)
            n272 = case shown="\"None\", Default" w731 {
              tunnel: [w738 State_Type_Definitions,_for_0.26g_versions_and_later_2."True Stop" ("Enum")] -> w729
              tunnel: [w737 w755] -> w728
              tunnel: [State_Type_Definitions,_for_0.26g_versions_and_later_2."Idle" ("Enum") State_Type_Definitions,_for_0.26g_versions_and_later_2."Shutdown" ("Enum")] -> w730
              tunnel: w727 -> [w733 _]
              tunnel: w723 -> [w735 _]
              tunnel: w721 -> [w732 _]
              frame "None", Default {
                n273 = case shown="False" w732 {
                  tunnel: [w743 w749] -> w737
                  tunnel: w735 -> [w741 w747]
                  frame False {
                    n274 = for {
                      tunnel: string[] ["Z STEPPER CAM HEIGHT", "READ STEPPER VALUES"] ("element") -> [w744] mode=indexing
                      shift-right: [w746] -> w743
                      shift-left: w741 -> [w745]
                      n275 = Enqueue Element(queue=w745, element=w744) -> (queue out=w746:refnum<queue>)  [unwired: 2 in, 2 out]
                    }
                  }
                  frame True {
                    n276 = for {
                      shift-right: [w751] -> w749
                      shift-left: w747 -> [w752]
                      tunnel: string[] ["CAM ACQ", ""] -> [w750] mode=indexing
                      n277 = Enqueue Element(queue=w752, element=w750) -> (queue out=w751:refnum<queue>)  [unwired: 2 in, 2 out]
                    }
                  }
                }
                n278 = Or(x=w732, y=w733) -> (x .or. y?=w734:bool)
                n279 = Select(t=State_Type_Definitions,_for_0.26g_versions_and_later_2."Task 6_B" ("Enum"), s=w734, f=State_Type_Definitions,_for_0.26g_versions_and_later_2."Task 6_A" ("Enum")) -> (s? t:f=w738:T6)
              }
              frame "Exit" {
                n280 = for {
                  shift-right: [w758] -> w755
                  shift-left: _ -> [w759]
                  tunnel: string[] ["STOP", "RESET ENCODERS", "RESET YAW", "ARDUINO MODE 0"] -> [w757] mode=indexing
                  n281 = Enqueue Element(queue=w759, element=w757) -> (queue out=w758:refnum<queue>)  [unwired: 2 in, 2 out]
                }
              }
            }
          }
          frame 24 {
            n282 = Dequeue Element(queue=w768, timeout in ms (-1)=w766, error in (no error)=w767) -> (element=w765:T7)  [unwired: 3 out]
            n283 = case shown="\"None\", Default" w765 {
              tunnel: [w775 State_Type_Definitions,_for_0.26g_versions_and_later_2."True Stop" ("Enum")] -> w761
              tunnel: [w774 w793] -> w769
              tunnel: [State_Type_Definitions,_for_0.26g_versions_and_later_2."Idle" ("Enum") State_Type_Definitions,_for_0.26g_versions_and_later_2."Shutdown" ("Enum")] -> w762
              tunnel: w764 -> [w770 _]
              tunnel: w763 -> [w772 _]
              tunnel: w760 -> [w771 w790]
              frame "None", Default {
                # ">> Manual override >>"
                n284 = case shown="True" w772 {
                  tunnel: [w780 w786] -> w774
                  tunnel: w771 -> [w779 w784]
                  frame False {
                    n285 = for {
                      shift-right: [w783] -> w780
                      shift-left: w779 -> [w782]
                      tunnel: string[] ["CAM ACQ", "OPEN CLAW"] -> [w781] mode=indexing
                      n286 = Enqueue Element(queue=w782, element=w781) -> (queue out=w783:refnum<queue>)  [unwired: 2 in, 2 out]
                    }
                  }
                  frame True {
                    n287 = for {
                      shift-right: [w788] -> w786
                      shift-left: w784 -> [w789]
                      tunnel: string[] ["CAM ACQ", "CLOSE CLAW"] -> [w787] mode=indexing
                      n288 = Enqueue Element(queue=w789, element=w787) -> (queue out=w788:refnum<queue>)  [unwired: 2 in, 2 out]
                    }
                  }
                }
                n289 = Select(t=State_Type_Definitions,_for_0.26g_versions_and_later_2."True Stop" ("Enum"), s=w770, f=State_Type_Definitions,_for_0.26g_versions_and_later_2."Task 6_B" ("Enum")) -> (s? t:f=w775:T6)
              }
              frame "Exit" {
                # ">> State after true stop >>"
                # ">> Goes to true stop >>"
                n290 = for {
                  shift-right: [w796] -> w793
                  shift-left: w790 -> [w797]
                  tunnel: string[] ["STOP", "RESET ENCODERS", "RESET YAW", ""] -> [w795] mode=indexing
                  n291 = Enqueue Element(queue=w797, element=w795) -> (queue out=w796:refnum<queue>)  [unwired: 2 in, 2 out]
                }
              }
            }
          }
        }
      }
    }
  }
  n292 = call <vilib>:"DIO Close.vi"("error in (no error)"=w23, "DIO Info In"=w26) -> ()  [unwired: 9 in, 1 out]
  n293 = call <vilib>:"DIO Close.vi"("error in (no error)"=w33, "DIO Info In"=w35) -> ()  [unwired: 9 in, 1 out]
  n294 = call <vilib>:"NavX Close.vi"("error in (no error)"=w4, "NavX Info In"=w3) -> ()  [unwired: 9 in, 1 out]
  n295 = call <vilib>:"DIO Close.vi"("error in (no error)"=w28, "DIO Info In"=w30) -> ()  [unwired: 9 in, 1 out]
  n296 = call <vilib>:"DIO Close.vi"("error in (no error)"=w11, "DIO Info In"=w12) -> ()  [unwired: 9 in, 1 out]
  n297 = call <vilib>:"DIO Close.vi"("error in (no error)"=w6, "DIO Info In"=w7) -> ()  [unwired: 9 in, 1 out]
  n298 = while {
    stop <- w1193 stop-if-true
    n299 = call <vilib>:"RT Get CPU Loads.vi"() -> ("CPU loads"=→"CPU loads":T5[])  [unwired: 10 in, 1 out]
    n300 = Wait (ms)(milliseconds to wait=u32 100) -> ()  [unwired: 1 out]
    n301 = call "FGV Bool.vi"("Init/Read/Write State"=States_for_Action_Engine."Read") -> ("Output node"=w1193:bool)  [unwired: 2 in, 1 out]
  }
  n302 = Merge Errors "Merge Errors"(w63, w62) -> (w45:errorcluster)
  n303 = Merge Errors(w49, w45) -> (w44:errorcluster)
  n304 = Destroy User Event(user event=w66, error in=w44) -> ()  [unwired: 1 out]
  n305 = Destroy User Event(user event=w67, error in=w44) -> ()  [unwired: 1 out]
  n306 = Unregister For Events(event registration refnum=w58, error in=w44) -> ()  [unwired: 1 out]
  n307 = Release Queue(queue=w40, error in (no error)=w44) -> (error out=w22:errorcluster)  [unwired: 1 in, 2 out]
  n308 = Release Queue(queue=w57, error in (no error)=w44) -> ()  [unwired: 1 in, 3 out]
  n309 = call <vilib>:"Simple Error Handler.vi"("error in (no error)"=w22) -> ("error out"=w21:errorcluster)  [unwired: 4 in, 4 out]
  n310 = call <vilib>:"Reset myRIO.vi"("error in (no error)"=w21) -> ("error out"=→"error out":errorcluster)  [unwired: 10 in]
